vi "Periodic Tasks.vi"(8 "error in":errorcluster) -> ()   [LabVIEW 2013]
doc: "This VI runs in parallel to other tasks. It can contain as many user-defined periodic loops as you need. These can carry out PID or other sorts of timed response."
uses:
  <vilib>/Rock Robotics/SystemInterfaces/Utilities/FPGA_UtilitiesLED Source.ctl
  <vilib>/Rock Robotics/SystemInterfaces/Utilities/FPGA_UtilitiesLED State.ctl
  <vilib>/Rock Robotics/WPI/DriverStation/WPI_DriverStationRobotMode2.ctl
  <vilib>/Platform/TimedLoop/XDataNode/timing_clust.ctl
  <vilib>/Platform/TimedLoop/XDataNode/nitl_modes.ctl
  <vilib>/Platform/TimedLoop/XDataNode/wakeup.ctl
  Robot Global Data.vi
  <vilib>/Rock Robotics/WPI/Solenoid/Deprecated/WPI_SolenoidSetBool.vi
  <vilib>/addons/control/pid/pid.llb/PID (DBL).vi
  <vilib>/Rock Robotics/WPI/Compressor/WPI_CompressorGetSetRefNum.vi
  <vilib>/Platform/TimedLoop/XDataNode/XDataNode.xnode
  <vilib>/Platform/TimedLoop/XDataNode/XDNodeRunTimeDep.lvlib
  <vilib>/addons/control/pid/NI_PID_pid.lvlib
  <vilib>/addons/control/pid/pid.llb/PID Control Input Filter (DBL).vi
  Encoder Values.ctl
panel:
  in  "Neutral Angle":dbl=25.8
  in  "Feed Angle":dbl=20.0
  in  "Full Court Angle":dbl=25.8
  in  "Pyramid Angle":dbl=31.0
  in  "Vision Angle":dbl=24.5
  in  "Full Court Main RPM":dbl=4000.0
  in  "Full Court Pre RPM":dbl=3500.0
  in  "Pyramid Main RPM":dbl=4000.0
  in  "Pyramid Pre RPM":dbl=3500.0
  in  "Vision Main RPM":dbl=4000.0
  in  "Vision Pre RPM":dbl=3500.0
  in  "Elevator Enabled":bool=TRUE
  in  "Two Disc Loading":bool=TRUE
  in  "Load Reverse Enabled":bool=TRUE
  in  "Load Roller Delay (ms)":dbl=250.0
  in  "Load Exit Delay (ms)":dbl=1000.0
  in  "Shoot Exit Delay (ms)":dbl=200.0
  out "RPM Ready":bool
  out "Elevator Neutral Enabled":bool
  out "Neutral Angle Ready":bool
  out "Feed Angle Ready":bool
  out "Auto Angle Enabled":bool
  in  "Elevator Angle":dbl
  in  "Elevator Pot Voltage":dbl
  out "Shoot Angle Ready":bool
  in  "Shooter Pre RPM":dbl
  in  "Shooter Main RPM":dbl
  in  "Shooter Pre Output":dbl
  in  "Shooter Main Output":dbl
  # "don't stop wheels before disc exits shooter"
  # "don't stop rollers before disc reaches hopper"
  # "reverse rollers to push discs\n(ensures ramp can lower in time)"
  # "reverse rollers to keep discs out\n(as opposed to simply stopping)"
  # "when IRs see 2 discs, reverse right roller"
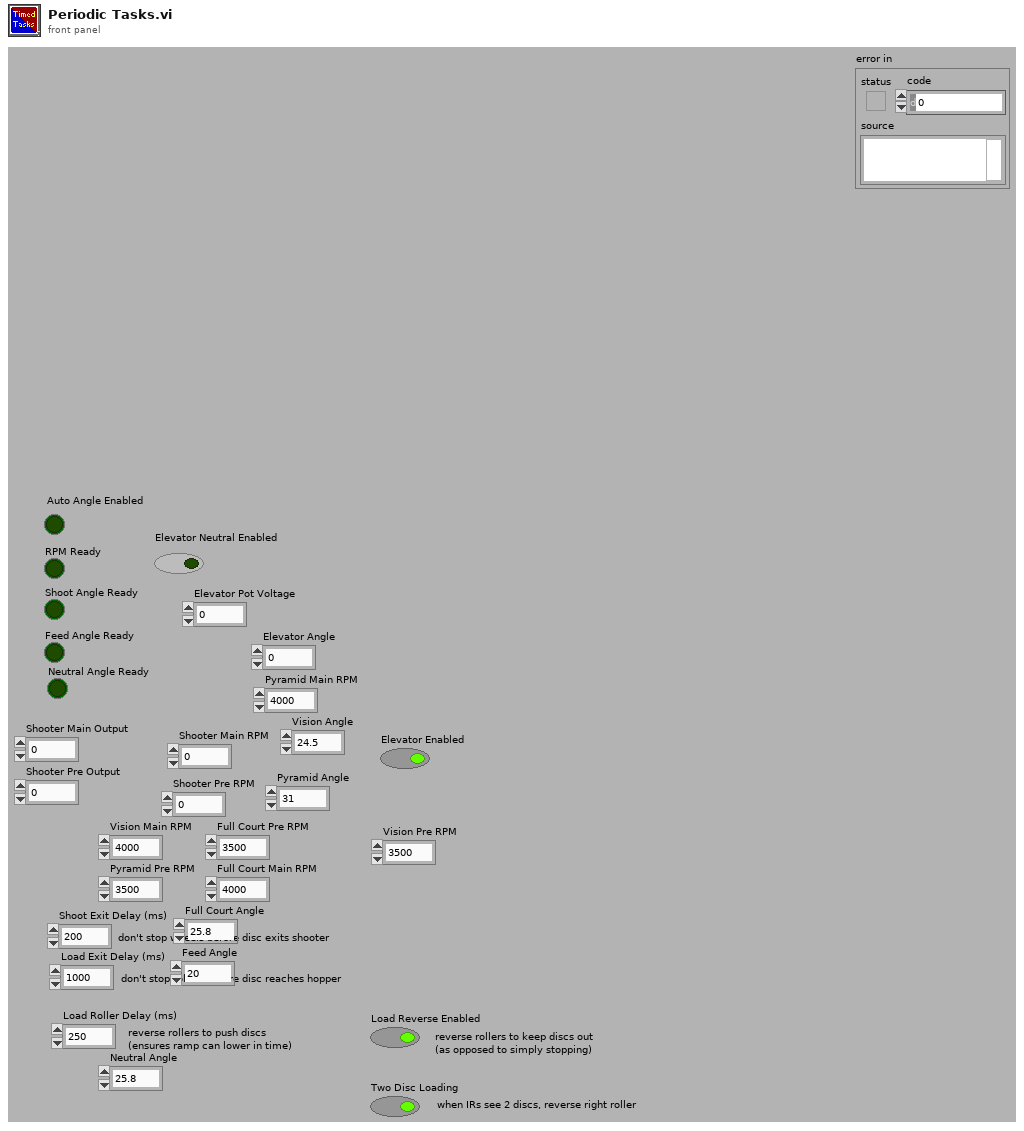
[diagram p1: front panel]
types:
  T1 = typedef "WPI_DriverStationRobotMode2.ctl" = enum16{"Autonomous Disabled", "Autonomous Enabled", "Teleop Disabled", "Teleop Enabled", "Timeout", "Finish", "Test Disabled", "Test Enabled"}
  T2 = enum16{"Vision", "Feed", "Pyramid", "Full Court"}
  T3 = cluster{"proportional gain (Kc)":dbl, "integral time (Ti, min)":dbl, "derivative time (Td, min)":dbl}
  T4 = typedef "Shoot Location.ctl" = enum16{"Vision", "Front", "Front Corner", "Back Corner", "Half Court", "Full Court", "Pyramid"}
  T5 = typedef "Autonomous Commands.ctl" = cluster{"Load":bool, "Warmup":bool, "Low Gear":bool, "Shoot Angle":dbl, "Azimuth":bool, "Elevator":bool, "Neutral Angle":dbl, "Two Discs":bool, "Shoot":bool}
  T6 = enum16{"Wait", "Adjust Angle", "Warmup Shooter", "Fire", "Feeding", "Neutral Angle"}
  T7 = typedef "XDNodeRunTimeDep.lvlib/timing_clust.ctl" = cluster{"Expected End [f-1]":u64, "Actual End [f-1]":u64, "Finished Late? [f-1]":bool, "Expected End [i-1]":u64, "Actual End [i-1]":u64, "Finished Late? [i-1]":bool, "Expected Start [i]":u64, "Actual Start [i]":u64, "Expected Start [f]":u64, "Actual Start [f]":u64, "Source Name":string, "Structure Name":string, "Period":i64, "Deadline":i64, "Offset":i64, "Start":i64, "Priority":i32, "Timeout":i32, "Mode":T8, "Wakeup Reason":T9, "Error":errorcluster, "Source Type":string, "Secondary Source Type":string, "Global End Time":u64, "Global Start Time":u64, "Frame Duration":u64, "Iteration Duration":u64, "Assigned CPU":i32, "I/O Scan Engine Mode":u32}
  T8 = typedef "XDNodeRunTimeDep.lvlib/nitl_modes.ctl" = enum32{"No Change", "Process missed periods, maintain original phase", "Discard missed periods, maintain original phase", "Process missed periods, ignore original phase", "Discard missed periods, ignore original phase"}
  T9 = typedef "XDNodeRunTimeDep.lvlib/wakeup.ctl" = enum32{"Normal", "Aborted", "Asynchronous wakeup", "Timing source error", "Timed loop error", "Timeout"}
  T10 = typedef "WPI_JoystickButtonState.ctl" = cluster{"Button 1":bool, "Button 2":bool, "Button 3":bool, "Button 4":bool, "Button 5":bool, "Button 6":bool, "Button 7":bool, "Button 8":bool, "Button 9":bool, "Button 10":bool, "Button 11":bool, "Button 12":bool}
  T11 = cluster{"Driver Axes":cluster{"axis 1 (x)":dbl, "axis 2 (y)":dbl, "axis 3 (throttle)":dbl, "axis 4":dbl, "axis 5":dbl, "axis 6":dbl}, "Driver Buttons":T10, "Manipulator Axes":cluster{"axis 1 (x)":dbl, "axis 2 (y)":dbl, "axis 3 (throttle)":dbl, "axis 4":dbl, "axis 5":dbl, "axis 6":dbl}, "Manipulator Buttons":T10}
  T12 = typedef "UDP Dashboard Packet.ctl" = cluster{"Feed Angle":dbl, "Neutral Angle":dbl, "Autonomous Setpoints":T13, "Auto Shift":T14, "Elevator Angle Offset":dbl, "Potentiometer Angle":cluster{"Pot M":dbl, "Pot B":dbl}, "Shoot Setpoints":cluster{"Vision":T15, "Back Corner":T15, "Front":T15, "Front Corner":T15, "Half Court":T15, "Full Court":T15, "Pyramid":T15}, "Halo Drive":T16, "Auto Speed Constants":T17, "Shooting Delays":cluster{"Unjam On":dbl, "Unjam Off":dbl, "Flipper On":dbl, "Flipper Off":dbl, "Hopper Up":dbl}, "Left Roller Pwr":dbl, "Right Roller Pwr":dbl, "Elevator PID Gains":cluster{"proportional gain (Kc)":dbl, "integral time (Ti, min)":dbl, "derivative time (Td, min)":dbl}, "Elevator PID Output Range":cluster{"output high":dbl, "output low":dbl}, "Elevator Angle Tolerance":dbl, "Toggle Ears Delay":dbl, "Toggle Ears Distance":dbl, "Unjam Servo Angle":dbl, "Auton Steer PID gains":cluster{"proportional gain (Kc)":dbl, "integral time (Ti, min)":dbl, "derivative time (Td, min)":dbl}, "Auton Steer output range":cluster{"output high":dbl, "output low":dbl}, "Auto Reverse Speed":dbl, "Auto Stop Throttle":dbl, "Auto Stop Duration":dbl, "Spin output range":cluster{"output high":dbl, "output low":dbl}, "Spin PID gains":cluster{"proportional gain (Kc)":dbl, "integral time (Ti, min)":dbl, "derivative time (Td, min)":dbl}, "Auto-Center Line":T18, "Auton Distance PID gains Low Gear":cluster{"proportional gain (Kc)":dbl, "integral time (Ti, min)":dbl, "derivative time (Td, min)":dbl}, "Auton Distance output range":cluster{"output high":dbl, "output low":dbl}, "Auton Distance Threshold":dbl, "Auton Velocity Cutoff":dbl, "Auton Distance output range Center Line":cluster{"output high":dbl, "output low":dbl}, "Auton Distance PID gains High Gear":cluster{"proportional gain (Kc)":dbl, "integral time (Ti, min)":dbl, "derivative time (Td, min)":dbl}}
  T13 = typedef "Autonomous Setpoints.ctl" = cluster{"Shoot Angle 1":dbl, "Initial Delay":dbl, "Disc Count 1":dbl, "Shoot Time 1":dbl, "Distance 1":dbl, "Two Disc Distance 1":dbl, "Distance 2":dbl, "Two Disc Distance 2":dbl, "Distance 3":dbl, "Two Disc Distance 3":dbl, "Shoot Angle 3":dbl, "Disc Count 3":dbl, "Shoot Time 3":dbl, "Distance 4":dbl, "Two Disc Distance 4":dbl, "Low Gear":bool, "Shoot 1 Post Delay":dbl}
  T14 = typedef "Auto Shift Settings.ctl" = cluster{"Enabled":bool, "Upshift Speed":dbl, "Downshift Speed":dbl, "Upshift Throttle":dbl, "Turn Power Diff":dbl, "Motor Limit":dbl, "Encoder Limit":dbl}
  T15 = typedef "Shoot Profile.ctl" = cluster{"Pre RPM":dbl, "Main RPM":dbl, "Angle":dbl}
  T16 = typedef "Halo Drive.ctl" = cluster{"Gains":cluster{"Quickturn_Sens_Low":dbl, "Quickturn_Sens_High":dbl, "Speedturn_Sens_Low":dbl, "Speedturn_Sens_High":dbl}, "QuickTurn Const":dbl, "Loading Throttle Limit":dbl}
  T17 = typedef "Auto Speed Constants.ctl" = cluster{"Slowing Distance":dbl, "High Speed":dbl, "Rampup Time":dbl, "Low Speed":dbl, "High Speed (Reverse)":dbl}
  T18 = typedef "Autonomous Center Line Setpoints.ctl" = cluster{"Arc Turn x-axis":dbl, "Arc Turn y-axis":dbl, "Arc Turn Distance":dbl, "Distance 1":dbl, "Two Disc Distance 1":dbl, "Distance 2":dbl, "Two Disc Distance 2":dbl, "Spin Angle":dbl, "Spin Angle tolerance":dbl, "Spin y-axis":dbl, "Spin Distance":dbl, "Center Line Enabled":bool, "Distance 3":dbl, "Two Disc Distance 3":dbl, "Spin Angle 2":dbl, "Spin Angle tolerance 2":dbl, "Spin y-axis 2":dbl, "Spin Distance 2":dbl, "Shoot Angle 1":dbl, "Disc Count 1":dbl, "Shoot Time 1":dbl, "Shoot Angle 3":dbl, "Disc Count 3":dbl, "Shoot Time 3":dbl, "Low Gear":bool}
  T19 = typedef "FPGA_UtilitiesLED State.ctl" = enum16{"Off", "On", "Toggle"}
  T20 = typedef "FPGA_UtilitiesLED Source.ctl" = enum16{"User LED", "FPGA LED"}
  T21 = typedef "WPI_CompressorDevRef.ctl" = cluster{"DevStatus":errorcluster, "DigitalInputDevRef":T22, "RelayDevRef":T25}
  T22 = typedef "WPI_DigitalInputDevRef.ctl" = cluster{"DevStatus":errorcluster, "DIO Channel":T23, "Digital Module":T24}
  T23 = typedef "FPGA_DIOChannel.ctl" = enum8{"DIO 1", "DIO 2", "DIO 3", "DIO 4", "DIO 5", "DIO 6", "DIO 7", "DIO 8", "DIO 9", "DIO 10", "DIO 11", "DIO 12", "DIO 13", "DIO 14", "Invalid"}
  T24 = typedef "FPGA_TypedefDigitalModule.ctl" = enum16{"Digital Module 1", "Digital Module 2"}
  T25 = typedef "WPI_RelayDevRef.ctl" = cluster{"DevStatus":errorcluster, "Relay Channel":T26, "Digital Module":T24, "Relay Direction":T27}
  T26 = typedef "FPGA_DIORelayChannel.ctl" = enum8{"Relay 1", "Relay 2", "Relay 3", "Relay 4", "Relay 5", "Relay 6", "Relay 7", "Relay 8", "Invalid"}
  T27 = typedef "WPI_RelayDirection.ctl" = enum16{"Both directions", "Forward only", "Reverse only"}
  T28 = typedef "WPI_GyroDevRef.ctl" = cluster{"DevStatus":errorcluster, "Analog Module":T29, "Analog Channel":T30, "Offset":dbl, "Gain (VoltsPerDegree/Second)":dbl}
  T29 = typedef "FPGA_TypedefAnalogModule.ctl" = enum16{"Analog Module 1", "Analog Module 2"}
  T30 = typedef "FPGA_AIChannel.ctl" = enum8{"AI 1", "AI 2", "AI 3", "AI 4", "AI 5", "AI 6", "AI 7", "AI 8", "Invalid"}
  T31 = typedef "WPI_EncoderDevRef.ctl" = cluster{"DevStatus":errorcluster, "EncoderIndex":T32, "CounterIndex":T33, "DistancePerCount":dbl, "Decoding Type":T34}
  T32 = typedef "FPGA_EncoderIdx.ctl" = enum8{"Enc 0", "Enc 1", "Enc 2", "Enc 3", "Invalid"}
  T33 = typedef "FPGA_CounterCtrSystemIndex.ctl" = enum8{"Ctr 0", "Ctr 1", "Ctr 2", "Ctr 3", "Ctr 4", "Ctr 5", "Ctr 6", "Ctr 7", "Invalid"}
  T34 = typedef "WPI_EncoderType.ctl" = enum16{"1x", "2x", "4x"}
  T35 = typedef "WPI_MotorControlDeviceRef.ctl" = cluster{"DeviceStatus":errorcluster, "Type":enum16{"PWM", "CAN"}, "PWM":cluster{"Digital Module":T24, "PWM Channel":T36, "DeadBand":T37}, "CAN":cluster{"Device Number":u8, "Control Mode":T38, "Semaphore":T39, "Max Vout":dbl}, "Invert":bool, "TransformRef":T40, "InvTransformRef":T40}
  T36 = typedef "FPGA_DIOPWMChannel.ctl" = enum8{"PWM 1", "PWM 2", "PWM 3", "PWM 4", "PWM 5", "PWM 6", "PWM 7", "PWM 8", "PWM 9", "PWM 10", "Invalid"}
  T37 = typedef "WPI_PWMDeadband.ctl" = cluster{"Name":string, "maxPositivePwm":i32, "minPositivePwm":i32, "centerPwm":i32, "maxNegativePwm":i32, "minNegativePwm":i32, "angularRange":u16}
  T38 = typedef "WPI_CANJaguar_ControlMode.ctl" = enum8{"Percent VBus", "Current", "Speed", "Position", "Voltage"}
  T39 = typedef "Semaphore RefNum" = refnum<k1>
  T40 = typedef "WPI_PWMTransform_ConPane.ctl" = refnum<vi>
  T41 = typedef "Encoder Values.ctl" = cluster{"Left Dist":dbl, "Left Speed":dbl, "Right Dist":dbl, "Right Speed":dbl, "Left Ticks":dbl, "Right Ticks":dbl, "Avg Distance":dbl, "Avg Speed":dbl}
  T42 = cluster{"Wheel IR 1":bool, "Wheel IR 2":bool, "Disc IR Front":bool, "Disc IR Front 2":bool, "Disc IR Hopper":bool, "Disc IR Shooter":bool}
  T43 = cluster{"axis 1 (x)":dbl, "axis 2 (y)":dbl, "axis 3 (throttle)":dbl, "axis 4":dbl, "axis 5":dbl, "axis 6":dbl}
  T44 = cluster{"Manual Unjam":bool, "Manual Flipper":bool}
  T45 = cluster{"Unjam On":dbl, "Unjam Off":dbl, "Flipper On":dbl, "Flipper Off":dbl, "Hopper Up":dbl}
  T46 = typedef "WPI_ServoDeviceRef.ctl" = cluster{"DeviceStatus":errorcluster, "Digital Module":T24, "PWM Channel":T36, "DeadBand":T37}
  T47 = cluster{"Throttle":dbl, "Wheel":dbl, "Right Motor":dbl, "Left Motor":dbl}
  T48 = typedef "WPI_SolenoidDevRef.ctl" = cluster{"DevStatus":errorcluster, "Solenoid Module":T49, "Forward Solenoid Channel":T50, "Reverse Solenoid Channel":T50}
  T49 = typedef "FPGA_TypedefSolenoidModule.ctl" = enum16{"Solenoid Module 1", "Solenoid Module 2"}
  T50 = typedef "WPI_SolenoidChannel.ctl" = enum8{"Solenoid 1", "Solenoid 2", "Solenoid 3", "Solenoid 4", "Solenoid 5", "Solenoid 6", "Solenoid 7", "Solenoid 8", "Invalid"}
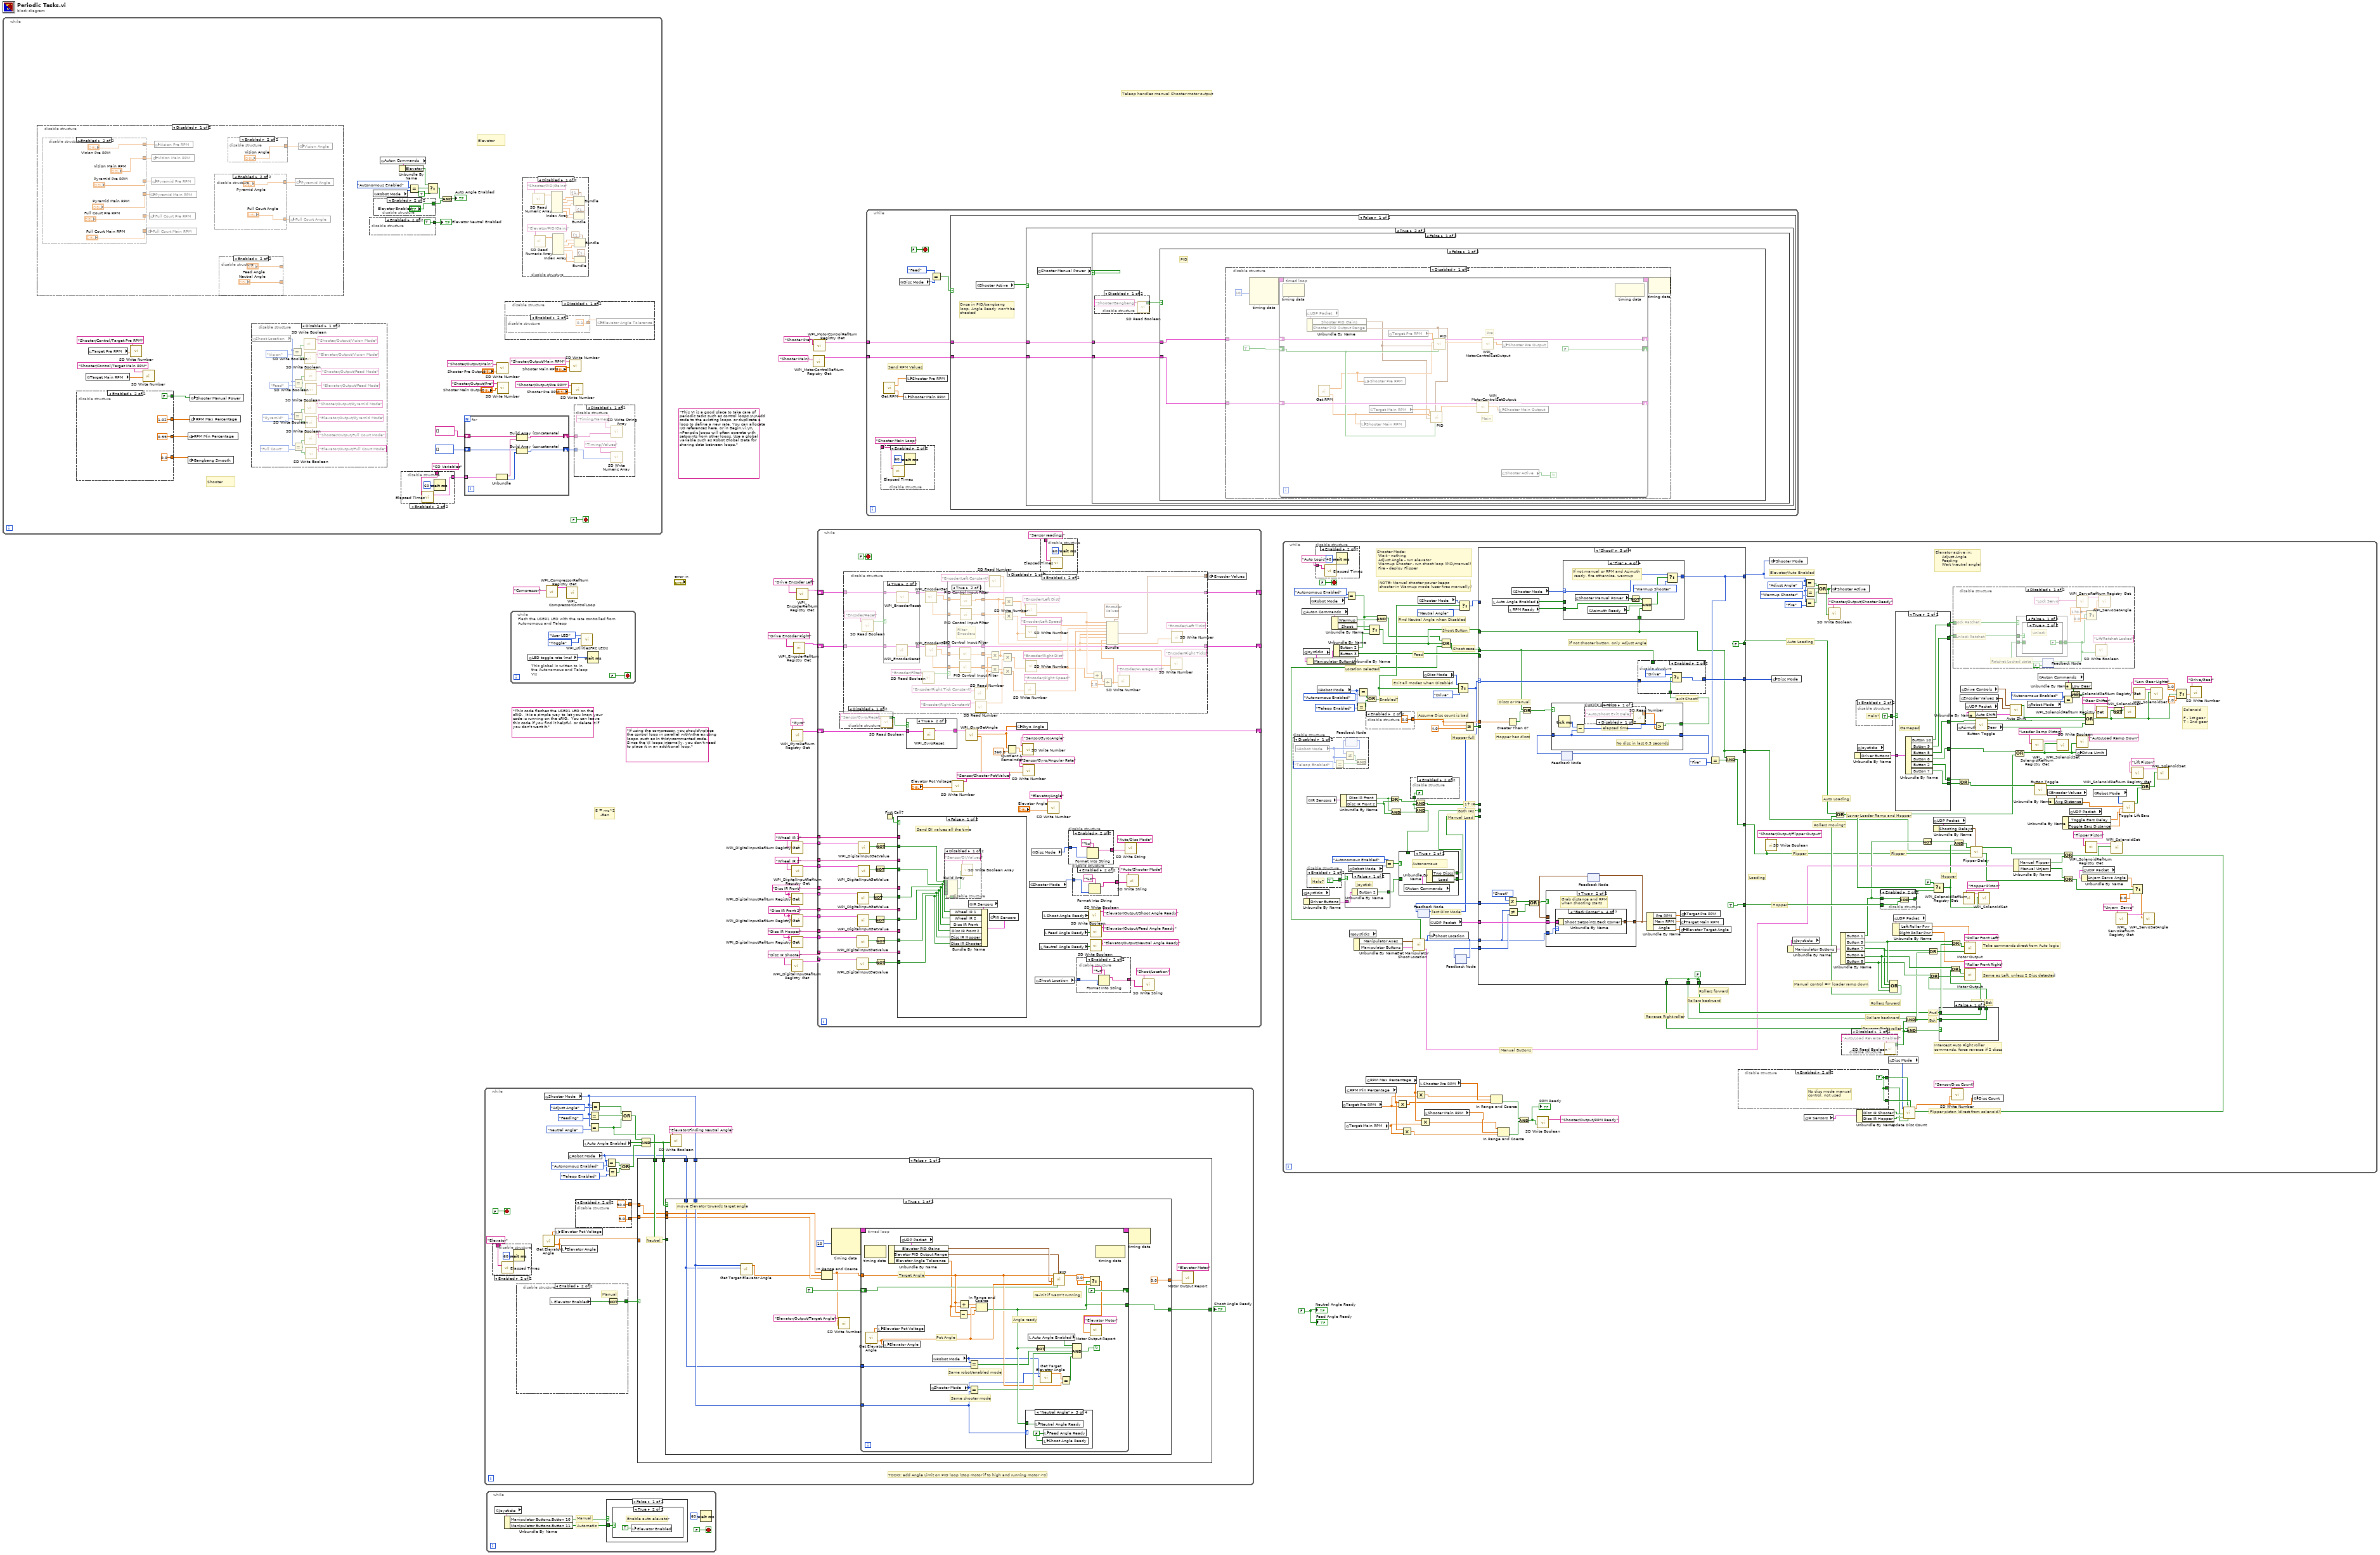
[diagram p0: block diagram]
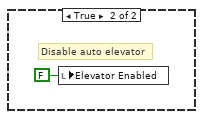
[diagram p3: hidden frame]
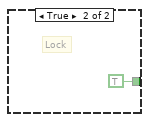
[diagram p5: hidden frame]
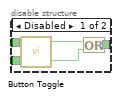
[diagram p7: hidden frame]
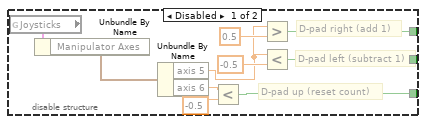
[diagram p9: hidden frame]
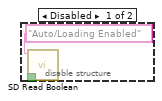
[diagram p10: hidden frame]
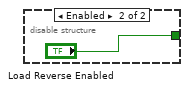
[diagram p11: hidden frame]
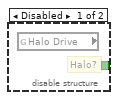
[diagram p12: hidden frame]
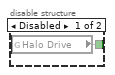
[diagram p13: hidden frame]
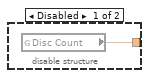
[diagram p15: hidden frame]
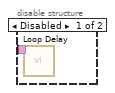
[diagram p16: hidden frame]
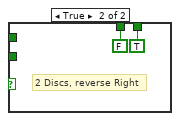
[diagram p17: hidden frame]
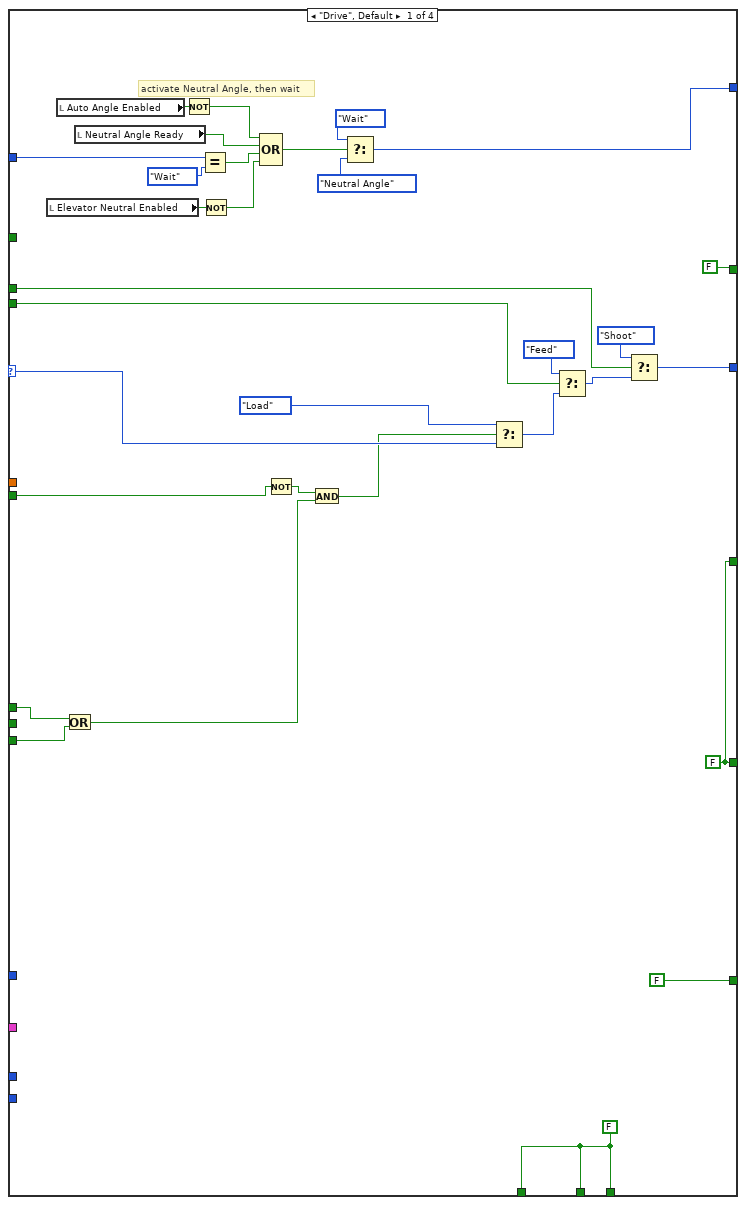
[diagram p18: hidden frame]
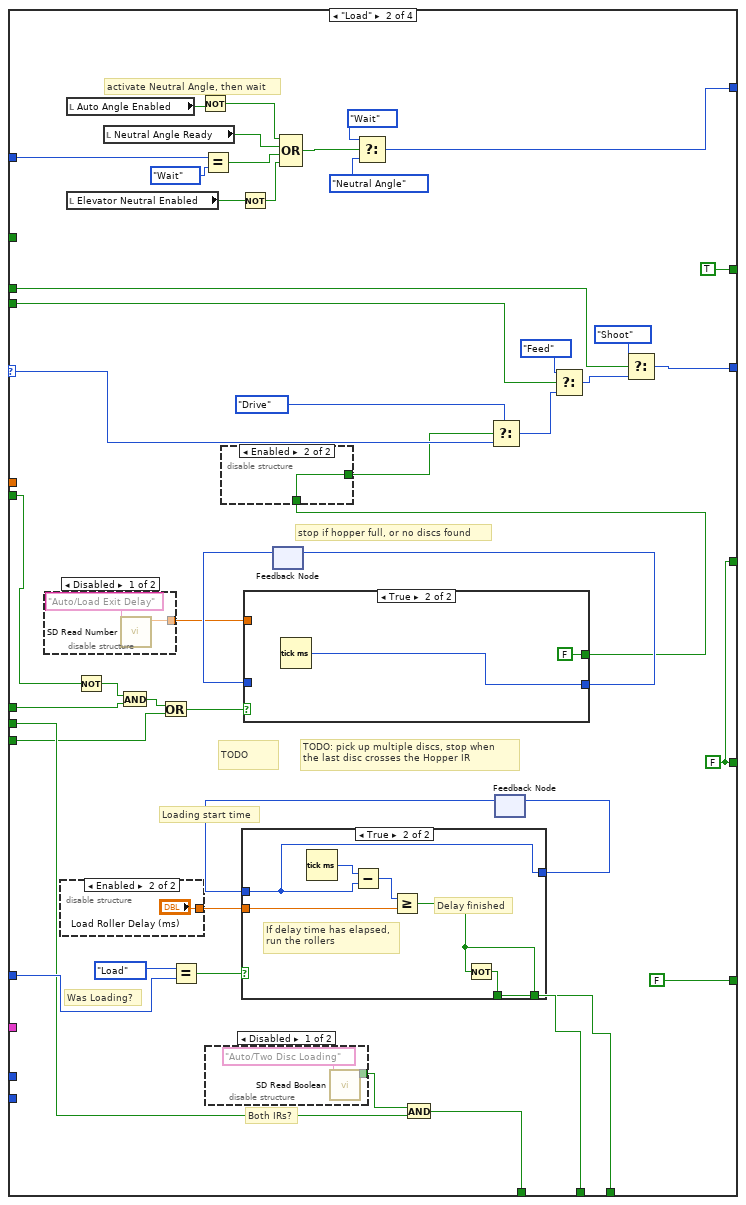
[diagram p19: hidden frame]
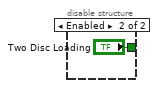
[diagram p20: hidden frame]
diagram:
  w1 = FALSE
  w2 = "Disc IR Shooter" ("refnum name")
  w6 = "Disc IR Hopper" ("refnum name")
  w5 = "Disc IR Front 2" ("refnum name")
  w4 = "Disc IR Front" ("refnum name")
  w11 = "Wheel IR 2" ("refnum name")
  w12 = "Wheel IR 1" ("refnum name")
  (unwired) "If using the compressor, you should\nplace the control loop in parallel with\nthe existing loops, such as in this\ncommented code. Since the VI loops internally, you don't need to place it in an additional loop."
  (unwired) "This code flashes the USER1 LED on the cRIO.  It is a simple way to let you know your code is running on the cRIO.  You can leave this code if you find it helpful, or delete it if you don't want it."
  (unwired) "This VI is a good place to take care of periodic tasks such as control loops.\n\nAdd code to the existing loops, or duplicate a loop to define a new rate. You can allocate I/O references here, or in Begin.vi.\n\nPeriodic loops will often operate with setpoints from other loops. Use a global variable such as Robot Global Data for sharing data between loops."
  # "Teleop handles manual Shooter motor output"
  # "E = mc^2\n    -Ben"
  n1 = while {
    stop <- FALSE stop-if-true
    # "Elevator"
    # "Shooter"
    n2 = disable-structure shown="Disabled" {
      frame Disabled {
        n3 = disable-structure shown="Enabled" {
          disable-tunnel: [w111 "Vision Pre RPM"] -> w88
          disable-tunnel: [w108 "Vision Main RPM"] -> w87
          disable-tunnel: [w107 "Pyramid Pre RPM"] -> w86
          disable-tunnel: [w104 "Pyramid Main RPM"] -> w85
          disable-tunnel: [w103 "Full Court Pre RPM"] -> w84
          disable-tunnel: [w100 "Full Court Main RPM"] -> w83
          frame Disabled {
            n4 = call <vilib>:"SD Read Number.vi"("Name"="Shooter/Control/Full Court Main RPM") -> ("Numeric"=w100:dbl)  [unwired: 8 in, 2 out]
            n5 = call <vilib>:"SD Read Number.vi"("Name"="Shooter/Control/Full Court Pre RPM") -> ("Numeric"=w103:dbl)  [unwired: 8 in, 2 out]
            n6 = call <vilib>:"SD Read Number.vi"("Name"="Shooter/Control/Vision Main RPM") -> ("Numeric"=w108:dbl)  [unwired: 8 in, 2 out]
            n7 = call <vilib>:"SD Read Number.vi"("Name"="Shooter/Control/Pyramid Pre RPM") -> ("Numeric"=w107:dbl)  [unwired: 8 in, 2 out]
            n8 = call <vilib>:"SD Read Number.vi"("Name"="Shooter/Control/Pyramid Main RPM") -> ("Numeric"=w104:dbl)  [unwired: 8 in, 2 out]
            n9 = call <vilib>:"SD Read Number.vi"("Name"="Shooter/Control/Vision Pre RPM") -> ("Numeric"=w111:dbl)  [unwired: 8 in, 2 out]
          }
          frame Enabled {
          }
        }
        n10 = global write "Robot Global Data.vi" "Full Court Main RPM"(w83) -> ()
        n11 = global write "Robot Global Data.vi" "Full Court Pre RPM"(w84) -> ()
        n12 = global write "Robot Global Data.vi" "Pyramid Main RPM"(w85) -> ()
        n13 = global write "Robot Global Data.vi" "Pyramid Pre RPM"(w86) -> ()
        n14 = global write "Robot Global Data.vi" "Vision Main RPM"(w87) -> ()
        n15 = global write "Robot Global Data.vi" "Vision Pre RPM"(w88) -> ()
        n16 = disable-structure shown="Enabled" {
          disable-tunnel: [w96 "Pyramid Angle"] -> w81
          disable-tunnel: [w95 "Full Court Angle"] -> w80
          frame Disabled {
            n17 = call <vilib>:"SD Read Number.vi"("Name"="Elevator/Full Court Angle") -> ("Numeric"=w95:dbl)  [unwired: 8 in, 2 out]
            n18 = call <vilib>:"SD Read Number.vi"("Name"="Elevator/Pyramid Angle") -> ("Numeric"=w96:dbl)  [unwired: 8 in, 2 out]
          }
          frame Enabled {
          }
        }
        n19 = disable-structure shown="Enabled" {
          disable-tunnel: [w121 "Feed Angle"] -> w90
          disable-tunnel: [w118 "Neutral Angle"] -> w89
          frame Disabled {
            n20 = call <vilib>:"SD Read Number.vi"("Name"="Elevator/Feed Angle") -> ("Numeric"=w121:dbl)  [unwired: 8 in, 2 out]
            n21 = call <vilib>:"SD Read Number.vi"("Name"="Elevator/Neutral Angle") -> ("Numeric"=w118:dbl)  [unwired: 8 in, 2 out]
          }
          frame Enabled {
          }
        }
        n22 = disable-structure shown="Enabled" {
          disable-tunnel: [w92 "Vision Angle"] -> w82
          frame Disabled {
            n23 = call <vilib>:"SD Read Number.vi"("Name"="Elevator/Vision Angle") -> ("Numeric"=w92:dbl)  [unwired: 8 in, 2 out]
          }
          frame Enabled {
          }
        }
        n24 = global write "Robot Global Data.vi" "Full Court Angle"(w80) -> ()
        n25 = global write "Robot Global Data.vi" "Pyramid Angle"(w81) -> ()
        n26 = global write "Robot Global Data.vi" "Vision Angle"(w82) -> ()
      }
      frame Enabled {
      }
    }
    n27 = disable-structure shown="Enabled" {
      disable-tunnel: [w136 0.0 ("Bangbang Smooth")] -> w52
      disable-tunnel: [w134 1.02 ("RPM Max Percentage")] -> w50
      disable-tunnel: [w133 0.99 ("RPM Min Percentage")] -> w49
      disable-tunnel: [w130 FALSE ("Shooter Manual Power")] -> w48
      frame Disabled {
        n28 = call <vilib>:"SD Read Number.vi"("Name"="Shooter/Control/RPM Min Percentage") -> ("Numeric"=w133:dbl)  [unwired: 8 in, 2 out]
        n29 = call <vilib>:"SD Read Number.vi"("Name"="Shooter/Bangbang Smooth") -> ("Numeric"=w136:dbl)  [unwired: 8 in, 2 out]
        n30 = call <vilib>:"SD Read Number.vi"("Name"="Shooter/Control/RPM Max Percentage") -> ("Numeric"=w134:dbl)  [unwired: 8 in, 2 out]
        n31 = call <vilib>:"SD Read Boolean.vi"("Name"="Shooter/Manual Power") -> ("Boolean"=w130:bool)  [unwired: 8 in, 2 out]
      }
      frame Enabled {
      }
    }
    n32 = global read "Robot Global Data.vi" "Target Main RPM"() -> (w27:dbl)
    n33 = global read "Robot Global Data.vi" "Target Pre RPM"() -> (w26:dbl)
    n34 = call <vilib>:"SD Write Number.vi"("Numeric"=w26, "Name"="Shooter/Control/Target Pre RPM") -> ()  [unwired: 8 in, 2 out]
    n35 = call <vilib>:"SD Write Number.vi"("Numeric"=w27, "Name"="Shooter/Control/Target Main RPM") -> ()  [unwired: 8 in, 2 out]
    n36 = global write "Robot Global Data.vi" "RPM Min Percentage"(w49) -> ()
    n37 = global write "Robot Global Data.vi" "Bangbang Smooth"(w52) -> ()
    n38 = global write "Robot Global Data.vi" "RPM Max Percentage"(w50) -> ()
    n39 = global write "Robot Global Data.vi" "Shooter Manual Power"(w48) -> ()
    n40 = disable-structure shown="Disabled" {
      frame Disabled {
        n41 = global read "Robot Global Data.vi" "Shoot Location"() -> (w67:T4)
        n42 = Equal?(x=w67, y=T2."Vision") -> (x = y?=w77:bool)
        n43 = Equal?(x=w67, y=T2."Pyramid") -> (x = y?=w71:bool)
        n44 = Equal?(x=w67, y=T2."Feed") -> (x = y?=w76:bool)
        n45 = Equal?(x=w67, y=T2."Full Court") -> (x = y?=w70:bool)
        n46 = call <vilib>:"SD Write Boolean.vi"("Boolean"=w77, "Name"="Shooter/Output/Vision Mode") -> ()  [unwired: 8 in, 2 out]
        n47 = call <vilib>:"SD Write Boolean.vi"("Boolean"=w77, "Name"="Elevator/Output/Vision Mode") -> ()  [unwired: 8 in, 2 out]
        n48 = call <vilib>:"SD Write Boolean.vi"("Boolean"=w71, "Name"="Shooter/Output/Pyramid Mode") -> ()  [unwired: 8 in, 2 out]
        n49 = call <vilib>:"SD Write Boolean.vi"("Boolean"=w76, "Name"="Shooter/Output/Feed Mode") -> ()  [unwired: 8 in, 2 out]
        n50 = call <vilib>:"SD Write Boolean.vi"("Boolean"=w70, "Name"="Shooter/Output/Full Court Mode") -> ()  [unwired: 8 in, 2 out]
        n51 = call <vilib>:"SD Write Boolean.vi"("Boolean"=w71, "Name"="Elevator/Output/Pyramid Mode") -> ()  [unwired: 8 in, 2 out]
        n52 = call <vilib>:"SD Write Boolean.vi"("Boolean"=w76, "Name"="Elevator/Output/Feed Mode") -> ()  [unwired: 8 in, 2 out]
        n53 = call <vilib>:"SD Write Boolean.vi"("Boolean"=w70, "Name"="Elevator/Output/Full Court Mode") -> ()  [unwired: 8 in, 2 out]
      }
      frame Enabled {
      }
    }
    n54 = disable-structure shown="Enabled" {
      disable-tunnel: [w127 TRUE ("Elevator Neutral Enabled")] -> w37
      frame Disabled {
        n55 = call <vilib>:"SD Read Boolean.vi"("Name"="Elevator/Neutral Enabled") -> ("Boolean"=w127:bool)  [unwired: 8 in, 2 out]
      }
      frame Enabled {
      }
    }
    "Elevator Neutral Enabled" <- w37
    n56 = global read "Robot Global Data.vi" "Robot Mode"() -> (w33:T1)
    n57 = disable-structure shown="Enabled" {
      disable-tunnel: [w124 "Elevator Enabled"] -> w35
      frame Disabled {
        n58 = call <vilib>:"SD Read Boolean.vi"("Name"="Elevator/Auto Enabled") -> ("Boolean"=w124:bool)  [unwired: 8 in, 2 out]
      }
      frame Enabled {
      }
    }
    n59 = global read "Robot Global Data.vi" "Auton Commands"() -> (w36:T5)
    n60 = Unbundle By Name(w36) -> ("Elevator"=w30:bool)
    n61 = disable-structure shown="Enabled" {
      disable-tunnel: "SD Variables" ("Call Name") -> [w165 w167]
      disable-tunnel: [w164 w166] -> w38
      frame Disabled {
        n62 = call "Loop Delay.vi"("Loop Name"=w165) -> ("Timings"=w164:cluster{"Call Name":string, "Delta (ms)":u32}[])  [unwired: 10 in]
      }
      frame Enabled {
        n63 = call "Elapsed Times.vi"("Call Name"=w167) -> ("Timings"=w166:cluster{"Call Name":string, "Delta (ms)":u32}[])  [unwired: 2 in]
        n64 = Wait (ms)(milliseconds to wait=u32 60 ("t")) -> ()  [unwired: 1 out]
      }
    }
    n65 = Equal?(x=WPI_DriverStationRobotMode2."Autonomous Enabled", y=w33) -> (x = y?=w31:bool)
    n66 = Select(t=w30, s=w31, f=TRUE) -> (s? t:f=w29:bool)
    n67 = And(x=w29, y=w35) -> (x .and. y?=→"Auto Angle Enabled":bool)
    n68 = for {
      tunnel: w38 -> [w175] mode=indexing
      shift-right: [w170] -> w55
      shift-left: string[] [] ("appended array") -> [w171]
      shift-right: [w169] -> w54
      shift-left: u32[] [] ("appended array") -> [w172]
      n69 = Unbundle(w175) -> ("Call Name"=w174:string, "Delta (ms)"=w173:u32)
      n70 = Build Array (concatenate)(w171, w174) -> (w170:string[])
      n71 = Build Array (concatenate)(w172, w173) -> (w169:u32[])
    }
    n72 = call <vilib>:"SD Write Number.vi"("Numeric"="Shooter Pre Output", "Name"="Shooter/Output/Main") -> ()  [unwired: 8 in, 2 out]
    n73 = call <vilib>:"SD Write Number.vi"("Numeric"="Shooter Main Output", "Name"="Shooter/Output/Pre") -> ()  [unwired: 8 in, 2 out]
    n74 = disable-structure shown="Disabled" {
      frame Disabled {
        n75 = disable-structure shown="Enabled" {
          disable-tunnel: [w60 0.1 ("Elevator Angle Tolerance")] -> w59
          frame Disabled {
            n76 = call <vilib>:"SD Read Number.vi"("Name"="Elevator/Control/Angle Tolerance") -> ("Numeric"=w60:dbl)  [unwired: 8 in, 2 out]
          }
          frame Enabled {
          }
        }
        n77 = global write "Robot Global Data.vi" "Elevator Angle Tolerance"(w59) -> ()
      }
      frame Enabled {
      }
    }
    n78 = disable-structure shown="Disabled" {
      frame Disabled {
        n79 = call <vilib>:"SD Read Numeric Array.vi"("Name"="Shooter/PID/Gains") -> ("Numeric Array"=w157:dbl[])  [unwired: 8 in, 2 out]
        n80 = call <vilib>:"SD Read Numeric Array.vi"("Name"="Elevator/PID/Gains") -> ("Numeric Array"=w148:dbl[])  [unwired: 8 in, 2 out]
        n81 = Index Array(array=w157) -> (element #1=w156:dbl, element #2=w155:dbl, element #3=w154:dbl, element #4=w143:dbl, element #5=w142:dbl)  [unwired: 5 in]
        n82 = Index Array(array=w148) -> (element #1=w149:dbl, element #2=w150:dbl, element #3=w151:dbl, element #4=w145:dbl, element #5=w144:dbl)  [unwired: 5 in]
        n83 = Bundle(cluster=cluster{"output high":dbl, "output low":dbl} {"output high"=100.0, "output low"=-100.0} ("output range"), "output high"=w143, "output low"=w142) -> ()  [unwired: 1 out]
        n84 = Bundle(cluster=T3 {"proportional gain (Kc)"=1.0, "integral time (Ti, min)"=0.01, "derivative time (Td, min)"=0.0} ("PID gains"), "proportional gain (Kc)"=w156, "integral time (Ti, min)"=w155, "derivative time (Td, min)"=w154) -> ()  [unwired: 1 out]
        n85 = Bundle(cluster=cluster{"output high":dbl, "output low":dbl} {"output high"=100.0, "output low"=-100.0} ("output range"), "output high"=w145, "output low"=w144) -> ()  [unwired: 1 out]
        n86 = Bundle(cluster=T3 {"proportional gain (Kc)"=1.0, "integral time (Ti, min)"=0.01, "derivative time (Td, min)"=0.0} ("PID gains"), "proportional gain (Kc)"=w149, "integral time (Ti, min)"=w150, "derivative time (Td, min)"=w151) -> ()  [unwired: 1 out]
      }
      frame Enabled {
      }
    }
    n87 = call <vilib>:"SD Write Number.vi"("Numeric"="Shooter Main RPM", "Name"="Shooter/Output/Main RPM") -> ()  [unwired: 8 in, 2 out]
    n88 = call <vilib>:"SD Write Number.vi"("Numeric"="Shooter Pre RPM", "Name"="Shooter/Output/Pre RPM") -> ()  [unwired: 8 in, 2 out]
    n89 = disable-structure shown="Disabled" {
      disable-tunnel: w55 -> [w163 _]
      disable-tunnel: w54 -> [w161 _]
      frame Disabled {
        n90 = call <vilib>:"SD Write String Array.vi"("String Array"=w163, "Name"="Timing/Names") -> ()  [unwired: 8 in, 2 out]
        n91 = call <vilib>:"SD Write Numeric Array.vi"("Numeric Array"=w161, "Name"="Timing/Values") -> ()  [unwired: 8 in, 2 out]
      }
      frame Enabled {
      }
    }
  }
  n92 = while {
    stop <- FALSE stop-if-true
    # "TODO: add Angle Limit on PID loop (stop motor if to high and running motor >0)"
    n93 = disable-structure shown="Enabled" {
      disable-tunnel: "Elevator" ("Call Name") -> [w215 w216]
      frame Disabled {
        n94 = call "Loop Delay.vi"("Loop Name"=w215) -> ()  [unwired: 10 in, 1 out]
      }
      frame Enabled {
        n95 = call "Elapsed Times.vi"("Call Name"=w216) -> ()  [unwired: 2 in, 1 out]
        n96 = Wait (ms)(milliseconds to wait=u32 60 ("t")) -> ()  [unwired: 1 out]
      }
    }
    n97 = disable-structure shown="Enabled" {
      disable-tunnel: [w202 w208] -> w198
      frame Disabled {
        # "Manual control button"
        n98 = global read "Robot Global Data.vi" "Joysticks"() -> (w200:T11)
        n99 = Unbundle By Name(w200) -> ("Manipulator Buttons.Button 10"=w202:bool, "Manipulator Buttons.Button 11"=w201:bool)
        n100 = case shown="True" w201 {
          frame False {
          }
          frame True {
            # "Enable auto elevator"
            n101 = disable-structure shown="Disabled" {
              disable-tunnel: TRUE ("Boolean") -> [w205 w206]
              frame Disabled {
                n102 = call <vilib>:"SD Write Boolean.vi"("Boolean"=w205, "Name"="Elevator/Auto Enabled") -> ()  [unwired: 8 in, 2 out]
              }
              frame Enabled {
                n103 = local write "Elevator Enabled"(w206) -> ()
              }
            }
          }
        }
      }
      frame Enabled {
        # "Manual"
        n104 = local read "Elevator Enabled"() -> (w207:bool)
        n105 = Not(x=w207) -> (.not. x?=w208:bool)
      }
    }
    n106 = call "Get Elevator Angle.vi"() -> ("Elevator Angle"=w196:dbl, "Pot Voltage"=w197:dbl)  [unwired: 2 in]
    n107 = global read "Robot Global Data.vi" "Shooter Mode"() -> (w191:T6)
    n108 = local write "Elevator Pot Voltage"(w197) -> ()
    n109 = local write "Elevator Angle"(w196) -> ()
    n110 = global read "Robot Global Data.vi" "Robot Mode"() -> (w176:T1)
    n111 = disable-structure shown="Enabled" {
      disable-tunnel: [w210 50.0 ("Numeric")] -> w195
      disable-tunnel: [w209 5.0 ("Numeric")] -> w194
      frame Disabled {
        n112 = call <vilib>:"SD Read Number.vi"("Name"="Elevator/Min Angle") -> ("Numeric"=w209:dbl)  [unwired: 8 in, 2 out]
        n113 = call <vilib>:"SD Read Number.vi"("Name"="Elevator/Max Angle") -> ("Numeric"=w210:dbl)  [unwired: 8 in, 2 out]
      }
      frame Enabled {
      }
    }
    n114 = local read "Auto Angle Enabled"() -> (w187:bool)
    n115 = Equal?(x=w191, y=T6."Feeding" ("Shooter Mode")) -> (x = y?=w192:bool)
    n116 = Equal?(x=w191, y=T6."Neutral Angle" ("Shooter Mode")) -> (x = y?=w177:bool)
    n117 = Equal?(x=w191, y=T6."Adjust Angle" ("Shooter Mode")) -> (x = y?=w193:bool)
    n118 = Equal?(x=w176, y=WPI_DriverStationRobotMode2."Autonomous Enabled") -> (x = y?=w183:bool)
    n119 = Equal?(x=w176, y=WPI_DriverStationRobotMode2."Teleop Enabled") -> (x = y?=w182:bool)
    n120 = Compound Arithmetic op=OR(w183, w182) -> (w181:bool)
    n121 = Compound Arithmetic op=OR(w193, w192, w177) -> (w188:bool)
    n122 = Compound Arithmetic op=AND(w188, w187, w181) -> (w186:bool)
    n123 = case shown="False" w198 {
      tunnel: [w221 TRUE] -> _
      tunnel: w196 -> [_ w290]
      tunnel: w195 -> [w220 w289]
      tunnel: w194 -> [w219 w291]
      tunnel: w186 -> [w223 _]
      tunnel: w191 -> [w224 _]
      tunnel: w177 -> [w222 _]
      tunnel: w176 -> [w218 _]
      frame False {
        # "Neutral"
        n124 = case shown="True" w223 {
          tunnel: [0.0 ("Numeric") 0.0 ("Numeric")] -> w226
          tunnel: [w238 TRUE] -> w221
          tunnel: w224 -> [w233 _]
          tunnel: w222 -> [_ _]
          tunnel: w220 -> [w231 _]
          tunnel: w219 -> [w230 _]
          tunnel: w218 -> [w229 _]
          frame True {
            # "move Elevator towards target angle"
            n125 = call "Get Target Elevator Angle.vi"("Robot Mode"=w229, "Shooter Mode"=w233) -> ("Target Angle"=w227:dbl)  [unwired: 9 in]
            n126 = In Range and Coerce(upper limit=w231, x=w227, lower limit=w230) -> (coerced(x)=w228:dbl)  [unwired: 1 out]
            n127 = node-c288(i64 10 ("Period")) -> (w237:T7)  [unwired: 2 in]
            n128 = call <vilib>:"SD Write Number.vi"("Numeric"=w228, "Name"="Elevator/Output/Target Angle") -> ()  [unwired: 8 in, 2 out]
            n129 = timed-loop {
              timing: w237 -> [_]
              timing-out: [_] -> w236
              shift-right: [FALSE ("x")] -> _
              shift-left: TRUE ("x") -> [w242]
              tunnel: w233 -> [w253]
              tunnel: [w256] -> w238
              tunnel: w228 -> [w247]
              tunnel: w229 -> [w251]
              stop <- w260 continue-if-true
              # "Same robot/enabled mode"
              # "Same shooter mode"
              # "Angle ready"
              # "re-init if wasn't running"
              # "Target Angle"
              # "Pot Angle"
              n130 = node-c288() -> ()  [unwired: 1 in, 1 out]
              n131 = call "Get Elevator Angle.vi"() -> ("Elevator Angle"=w259:dbl, "Pot Voltage"=w264:dbl)  [unwired: 2 in]
              n132 = local write "Elevator Pot Voltage"(w264) -> ()
              n133 = local write "Elevator Angle"(w259) -> ()
              n134 = global read "Robot Global Data.vi" "UDP Packet"() -> (w244:T12)
              n135 = Unbundle By Name(w244) -> ("Elevator PID Gains"=w243:T3, "Elevator PID Output Range"=w241:cluster{"output high":dbl, "output low":dbl}, "Elevator Angle Tolerance"=w240:dbl)
              n136 = global read "Robot Global Data.vi" "Shooter Mode"() -> (w245:T6)
              n137 = global read "Robot Global Data.vi" "Robot Mode"() -> (w246:T1)
              n138 = Subtract(x=w247, y=w240) -> (x-y=w257:dbl)
              n139 = Add(x=w247, y=w240) -> (x+y=w258:dbl)
              n140 = Equal?(x=w246, y=w251) -> (x = y?=w250:bool)
              n141 = Equal?(x=w245, y=w253) -> (x = y?=w252:bool)
              n142 = In Range and Coerce(upper limit=w258, x=w259, lower limit=w257) -> (In Range?=w256:bool)  [unwired: 1 out]
              n143 = case shown="\"Neutral Angle\"" w253 {
                tunnel: w256 -> [w268 w270 w272 _]
                frame "Adjust Angle" {
                  w267 = FALSE
                  n144 = local write "Shoot Angle Ready"(w268) -> ()
                  n145 = local write "Neutral Angle Ready"(w267) -> ()
                  n146 = local write "Feed Angle Ready"(w267) -> ()
                }
                frame "Feeding" {
                  w269 = FALSE
                  n147 = local write "Feed Angle Ready"(w270) -> ()
                  n148 = local write "Neutral Angle Ready"(w269) -> ()
                  n149 = local write "Shoot Angle Ready"(w269) -> ()
                }
                frame "Neutral Angle" {
                  w271 = FALSE
                  n150 = local write "Neutral Angle Ready"(w272) -> ()
                  n151 = local write "Shoot Angle Ready"(w271) -> ()
                  n152 = local write "Feed Angle Ready"(w271) -> ()
                }
                frame Default {
                }
              }
              n153 = local read "Auto Angle Enabled"() -> (w254:bool)
              n154 = Not(x=w256) -> (.not. x?=w255:bool)
              n155 = call "Get Target Elevator Angle.vi"("Robot Mode"=w246, "Shooter Mode"=w245) -> ("Target Angle"=w248:dbl)  [unwired: 9 in]
              n156 = call-poly <vilib>:"PID.vi"("reinitialize? (F)"=w242, "output range"=w241, "PID gains"=w243, "process variable"=w259, "setpoint"=w247) -> ("output"=w266:dbl)  [unwired: 5 in, 1 out]
              n157 = Equal?(x=w248, y=w247) -> (x = y?=w249:bool)
              n158 = Compound Arithmetic op=AND(w254, w255, w250, w252, w249) -> (w260:bool)
              n159 = Select(t=0.0, s=w256, f=w266) -> (s? t:f=w262:dbl)
              n160 = call "Motor Output Report.vi"("Motor Speed"=w262, "Motor refnum name"="Elevator Motor" ("refnum name")) -> ()  [unwired: 9 in, 1 out]
              n161 = node-c288() -> ()  [unwired: 1 in, 1 out]
            }
            n162 = node-c288(w236) -> ()  [unwired: 1 out]
          }
          frame False {
            # "Elevator not active"
          }
        }
        n163 = call "Motor Output Report.vi"("Motor Speed"=w226, "Motor refnum name"="Elevator Motor" ("refnum name")) -> ()  [unwired: 9 in, 1 out]
      }
      frame True {
        # "Manual"
        # "Within lower limit"
        # "Within upper limit"
        # "Manual override button"
        n164 = global read "Robot Global Data.vi" "Joysticks"() -> (w285:T11)
        n165 = Unbundle By Name(w285) -> ("Manipulator Buttons.Button 10"=w282:bool)
        n166 = global read "Robot Global Data.vi" "Joysticks"() -> (w286:T11)
        n167 = Greater?(x=w289, y=w290) -> (0:w288:bool)
        n168 = Unbundle By Name(w286) -> ("Manipulator Axes.axis 2 (y)"=w296:dbl)
        n169 = Less?(x=w291, y=w290) -> (x < y?=w287:bool)
        n170 = disable-structure shown="Disabled" {
          frame Disabled {
            # "Disable auto elevator"
            n171 = disable-structure shown="Enabled" {
              disable-tunnel: FALSE ("Boolean") -> [w298 w300]
              frame Disabled {
                n172 = call <vilib>:"SD Write Boolean.vi"("Boolean"=w298, "Name"="Elevator/Auto Enabled") -> ()  [unwired: 8 in, 2 out]
              }
              frame Enabled {
                n173 = local write "Elevator Enabled"(w300) -> ()
              }
            }
          }
          frame Enabled {
          }
        }
        n174 = Negate(x=w296) -> (-x=w284:dbl)
        n175 = disable-structure shown="Disabled" {
          disable-tunnel: [w302 TRUE ("Boolean")] -> w294
          frame Disabled {
            n176 = call <vilib>:"SD Read Boolean.vi"("Name"="Motor/Control/Elevator Analog") -> ("Boolean"=w302:bool)  [unwired: 8 in, 2 out]
          }
          frame Enabled {
            # "Elevator Analog"
          }
        }
        n177 = Select(t=w284, s=w282, f=0.0) -> (s? t:f=w283:dbl)
        n178 = call "Joystick Filter.vi"("In"=w283) -> ("Out"=w293:dbl)
        n179 = case shown="True" w294 {
          tunnel: "Elevator Motor" ("refnum name") -> [w312 w320]
          tunnel: w293 -> [w311 w318]
          tunnel: w288 -> [w306 w317]
          tunnel: w287 -> [w305 w319]
          frame False {
            # "Toggle motors"
            n180 = Greater Or Equal?(x=w311, y=0.5) -> (x >= y?=w308:bool)
            n181 = Less Or Equal?(x=w311, y=-0.5) -> (x <= y?=w310:bool)
            n182 = And(x=w305, y=w310) -> (x .and. y?=w309:bool)
            n183 = And(x=w308, y=w306) -> (x .and. y?=w307:bool)
            n184 = call "Motor Output.vi"("Max Power"=1.0, "Backward"=w309, "Forward"=w307, "Motor refnum name"=w312) -> ()  [unwired: 7 in, 1 out]
          }
          frame True {
            # "Joystick to motors"
            n185 = case shown="False" w319 {
              tunnel: w318 -> [w327 w328]
              tunnel: [w325 w328] -> w316
              frame False {
                # "Angle too LOW \nLimit power >0"
                n186 = Max & Min(x=0.0, y=w327) -> (max(x,y)=w325:dbl)  [unwired: 1 out]
              }
              frame True {
                # "Angle not too low"
              }
            }
            n187 = case shown="False" w317 {
              tunnel: w316 -> [w323 w324]
              tunnel: [w321 w324] -> w315
              frame False {
                # "Angle too HIGH\nLimit power <0"
                n188 = Max & Min(x=0.0, y=w323) -> (min(x,y)=w321:dbl)  [unwired: 1 out]
              }
              frame True {
                # "Angle not too high"
              }
            }
            n189 = call "Motor Output Report.vi"("Motor Speed"=w315, "Motor refnum name"=w320) -> ()  [unwired: 9 in, 1 out]
          }
        }
      }
    }
    n190 = call <vilib>:"SD Write Boolean.vi"("Boolean"=w186, "Name"="Elevator/Finding Neutral Angle") -> ()  [unwired: 8 in, 2 out]
  }
  n191 = while {
    stop <- FALSE stop-if-true
    # "Automatic"
    # "Manual"
    n192 = global read "Robot Global Data.vi" "Joysticks"() -> (w333:T11)
    n193 = Unbundle By Name(w333) -> ("Manipulator Buttons.Button 10"=w330:bool, "Manipulator Buttons.Button 11"=w329:bool)
    n194 = case shown="False" w330 {
      tunnel: w329 -> [w334 _]
      frame False {
        n195 = case shown="True" w334 {
          frame False {
          }
          frame True {
            # "Enable auto elevator"
            n196 = local write "Elevator Enabled"(TRUE ("Boolean")) -> ()
          }
        }
      }
      frame True {
        # "Disable auto elevator"
        n197 = local write "Elevator Enabled"(FALSE ("Boolean")) -> ()
      }
    }
    n198 = Wait (ms)(milliseconds to wait=u32 60) -> ()  [unwired: 1 out]
  }
  n199 = while {
    stop <- FALSE stop-if-true
    # "This global is written to in the Autonomous and Teleop VIs"
    # "Flash the USER1 LED with the rate controlled from Autonomous and Teleop"
    n200 = global read "Robot Global Data.vi" "LED toggle rate (ms)"() -> (w337:u32)
    n201 = call <vilib>:"WPI_UtilitiesFRC LEDs.vi"("State"=FPGA_UtilitiesLED_State."Toggle", "LED Type"=FPGA_UtilitiesLED_Source."User LED") -> ()  [unwired: 1 in, 9 out]
    n202 = Wait (ms)(milliseconds to wait=w337) -> ()  [unwired: 1 out]
  }
  n203 = call <vilib>:"WPI_CompressorRefNum Registry Get.vi"("refnum name"="Compressor") -> ("CompressorDevRef"=w25:T21)  [unwired: 9 in, 1 out]
  n204 = call <vilib>:"WPI_CompressorControlLoop.vi"("CompressorDevRef"=w25) -> ()  [unwired: 11 in]
  n205 = call <vilib>:"WPI_DigitalInputRefNum Registry Get.vi"("refnum name"=w2) -> ("DigitalInputDevRef"=w3:T22)  [unwired: 9 in, 1 out]
  n206 = call <vilib>:"WPI_GyroRefNum Registry Get.vi"("refnum name"="Gyro") -> ("GyroDevRef"=w18:T28)  [unwired: 9 in, 1 out]
  n207 = call <vilib>:"WPI_DigitalInputRefNum Registry Get.vi"("refnum name"=w12) -> ("DigitalInputDevRef"=w17:T22)  [unwired: 9 in, 1 out]
  n208 = call <vilib>:"WPI_DigitalInputRefNum Registry Get.vi"("refnum name"=w11) -> ("DigitalInputDevRef"=w16:T22)  [unwired: 9 in, 1 out]
  n209 = call <vilib>:"WPI_DigitalInputRefNum Registry Get.vi"("refnum name"=w4) -> ("DigitalInputDevRef"=w15:T22)  [unwired: 9 in, 1 out]
  n210 = call <vilib>:"WPI_DigitalInputRefNum Registry Get.vi"("refnum name"=w5) -> ("DigitalInputDevRef"=w14:T22)  [unwired: 9 in, 1 out]
  n211 = call <vilib>:"WPI_DigitalInputRefNum Registry Get.vi"("refnum name"=w6) -> ("DigitalInputDevRef"=w13:T22)  [unwired: 9 in, 1 out]
  n212 = call <vilib>:"WPI_EncoderRefNum Registry Get.vi"("refnum name"="Drive Encoder Right") -> ("EncoderDevRef"=w20:T31)  [unwired: 9 in, 1 out]
  n213 = call <vilib>:"WPI_EncoderRefNum Registry Get.vi"("refnum name"="Drive Encoder Left") -> ("EncoderDevRef"=w21:T31)  [unwired: 9 in, 1 out]
  n214 = call <vilib>:"WPI_MotorControlRefNum Registry Get.vi"("refnum name"="Shooter Main") -> ("MotorControlDevRef"=w9:T35)  [unwired: 9 in, 1 out]
  n215 = call <vilib>:"WPI_MotorControlRefNum Registry Get.vi"("refnum name"="Shooter Pre") -> ("MotorControlDevRef"=w7:T35)  [unwired: 9 in, 1 out]
  n216 = while {
    shift-right: [w351] -> _
    shift-left: w21 -> [w364]
    shift-right: [w350] -> _
    shift-left: w20 -> [w400]
    shift-right: [w392] -> _
    shift-left: w18 -> [w397]
    tunnel: w17 -> [w388]
    tunnel: w16 -> [w387]
    tunnel: w15 -> [w386]
    tunnel: w14 -> [w385]
    tunnel: w13 -> [w384]
    tunnel: w12 -> [w383]
    tunnel: w11 -> [w382]
    tunnel: w4 -> [w381]
    tunnel: w5 -> [w380]
    tunnel: w6 -> [w379]
    tunnel: w3 -> [w378]
    tunnel: w2 -> [w377]
    stop <- FALSE stop-if-true
    n217 = disable-structure shown="Disabled" {
      disable-tunnel: [w428 FALSE ("Boolean")] -> w396
      frame Disabled {
        n218 = call <vilib>:"SD Read Boolean.vi"("Name"="Sensor/Gyro/Reset") -> ("Boolean"=w428:bool)  [unwired: 8 in, 2 out]
      }
      frame Enabled {
        # "Reset gryo"
      }
    }
    n219 = disable-structure shown="Disabled" {
      disable-tunnel: w400 -> [w467 w500]
      disable-tunnel: [w466 w496] -> w399
      disable-tunnel: w364 -> [w464 w501]
      disable-tunnel: [w457 w499] -> w351
      disable-tunnel: [w456 w498] -> w350
      frame Disabled {
        n220 = call <vilib>:"SD Read Boolean.vi"("Name"="Encoder/Reset") -> ("Boolean"=w463:bool)  [unwired: 8 in, 2 out]
        n221 = case shown="True" w463 {
          tunnel: w467 -> [w491 w495]
          tunnel: [w491 w494] -> w472
          tunnel: [w490 w493] -> w465
          tunnel: w464 -> [w490 w492]
          frame False {
          }
          frame True {
            n222 = call <vilib>:"WPI_EncoderReset.vi"("EncoderDevRef"=w495) -> ("EncoderDevRef"=w494:T31)  [unwired: 9 in, 1 out]
            n223 = call <vilib>:"WPI_EncoderReset.vi"("EncoderDevRef"=w492) -> ("EncoderDevRef"=w493:T31)  [unwired: 9 in, 1 out]
          }
        }
        n224 = call <vilib>:"SD Read Boolean.vi"("Name"="Encoder/Filter") -> ("Boolean"=w450:bool)  [unwired: 8 in, 2 out]
        n225 = call <vilib>:"WPI_EncoderGet.vi"("EncoderDevRef"=w465) -> ("Distance"=w454:dbl, "EncoderDevRef"=w459:T31, "Rate"=w455:dbl)  [unwired: 5 in, 3 out]
        n226 = call <vilib>:"WPI_EncoderGet.vi"("EncoderDevRef"=w472) -> ("Distance"=w453:dbl, "EncoderDevRef"=w458:T31, "Rate"=w452:dbl)  [unwired: 5 in, 3 out]
        n227 = case shown="True" w450 {
          tunnel: w459 -> [w479 w489]
          tunnel: w458 -> [w476 w488]
          tunnel: [w479 w489] -> w457
          tunnel: [w476 w488] -> w456
          tunnel: w454 -> [w478 w487]
          tunnel: w455 -> [w477 w486]
          tunnel: [w477 w485] -> w449
          tunnel: [w478 w484] -> w432
          tunnel: w452 -> [w474 w483]
          tunnel: w453 -> [w475 w482]
          tunnel: [w475 w481] -> w437
          tunnel: [w474 w480] -> w440
          frame False {
            # "No filtering"
          }
          frame True {
            # "Filter\nEncoders"
            n228 = call-poly <vilib>:"PID Control Input Filter.vi"("input"=w482) -> ("output"=w481:dbl)  [unwired: 4 in]
            n229 = call-poly <vilib>:"PID Control Input Filter.vi"("input"=w483) -> ("output"=w480:dbl)  [unwired: 4 in]
            n230 = call-poly <vilib>:"PID Control Input Filter.vi"("input"=w487) -> ("output"=w484:dbl)  [unwired: 4 in]
            n231 = call-poly <vilib>:"PID Control Input Filter.vi"("input"=w486) -> ("output"=w485:dbl)  [unwired: 4 in]
          }
        }
        n232 = call <vilib>:"SD Read Number.vi"("Name"="Encoder/Right Tick Constant") -> ("Numeric"=w438:dbl)  [unwired: 8 in, 2 out]
        n233 = call <vilib>:"SD Read Number.vi"("Name"="Encoder/Right Constant") -> ("Numeric"=w441:dbl)  [unwired: 8 in, 2 out]
        n234 = call <vilib>:"SD Read Number.vi"("Name"="Encoder/Left Constant") -> ("Numeric"=w444:dbl)  [unwired: 8 in, 2 out]
        n235 = Multiply(x=w437, y=w438) -> (x*y=w433:dbl)
        n236 = Multiply(x=w440, y=w438) -> (x*y=w439:dbl)
        n237 = Multiply(x=w433, y=w441) -> (x*y=w434:dbl)
        n238 = Multiply(x=w439, y=w441) -> (x*y=w448:dbl)
        n239 = Multiply(x=w432, y=w444) -> (x*y=w446:dbl)
        n240 = Multiply(x=w449, y=w444) -> (x*y=w447:dbl)
        n241 = call <vilib>:"SD Write Number.vi"("Numeric"=w448, "Name"="Encoder/Right Speed") -> ()  [unwired: 8 in, 2 out]
        n242 = call <vilib>:"SD Write Number.vi"("Numeric"=w446, "Name"="Encoder/Left Dist") -> ()  [unwired: 8 in, 2 out]
        n243 = call <vilib>:"SD Write Number.vi"("Numeric"=w447, "Name"="Encoder/Left Speed") -> ()  [unwired: 8 in, 2 out]
        n244 = call <vilib>:"SD Write Number.vi"("Numeric"=w434, "Name"="Encoder/Right Dist") -> ()  [unwired: 8 in, 2 out]
        n245 = Add(x=w446, y=w434) -> (x+y=w461:dbl)
        n246 = Divide(x=w461, y=2.0) -> (x/y=w430:dbl)
        n247 = Bundle(cluster=T41 {"Left Dist"=-0.6624599999999999, "Left Speed"=0.0, "Right Dist"=-0.6850325099999999, "Right Speed"=0.0, "Left Ticks"=-91.5, "Right Ticks"=-94.61774999999999, "Avg Distance"=-94.61774999999999, "Avg Speed"=0.0} ("output cluster"), "Left Dist"=w446, "Left Speed"=w447, "Right Dist"=w434, "Right Speed"=w448, "Left Ticks"=w432, "Right Ticks"=w433, "Avg Distance"=w430) -> (w466:T41)  [unwired: 1 in]
        n248 = call <vilib>:"SD Write Number.vi"("Numeric"=w430, "Name"="Encoder/Average Dist") -> ()  [unwired: 8 in, 2 out]
        n249 = call <vilib>:"SD Write Number.vi"("Numeric"=w433, "Name"="Encoder/Right Ticks") -> ()  [unwired: 8 in, 2 out]
        n250 = call <vilib>:"SD Write Number.vi"("Numeric"=w432, "Name"="Encoder/Left Ticks") -> ()  [unwired: 8 in, 2 out]
      }
      frame Enabled {
        n251 = call "Read Encoders.vi"("Reset"=FALSE, "Right Encoder"=w500, "Left Encoder"=w501) -> ("Encoder Values"=w496:T41, "Right Encoder Out"=w498:T31, "Left Encoder Out"=w499:T31)  [unwired: 6 in]
      }
    }
    n252 = call <vilib>:"WPI_DigitalInputGetValue.vi"("DigitalInputDevRef"=w378) -> ("Value"=w376:bool)  [unwired: 8 in, 2 out]
    n253 = call <vilib>:"WPI_DigitalInputGetValue.vi"("DigitalInputDevRef"=w384) -> ("Value"=w373:bool)  [unwired: 8 in, 2 out]
    n254 = call <vilib>:"WPI_DigitalInputGetValue.vi"("DigitalInputDevRef"=w386) -> ("Value"=w370:bool)  [unwired: 8 in, 2 out]
    n255 = call <vilib>:"WPI_DigitalInputGetValue.vi"("DigitalInputDevRef"=w385) -> ("Value"=w372:bool)  [unwired: 8 in, 2 out]
    n256 = call <vilib>:"WPI_DigitalInputGetValue.vi"("DigitalInputDevRef"=w387) -> ("Value"=w368:bool)  [unwired: 8 in, 2 out]
    n257 = call <vilib>:"WPI_DigitalInputGetValue.vi"("DigitalInputDevRef"=w388) -> ("Value"=w366:bool)  [unwired: 8 in, 2 out]
    n258 = Not(x=w370) -> (.not. x?=w369:bool)
    n259 = Not(x=w368) -> (.not. x?=w367:bool)
    n260 = Not(x=w372) -> (.not. x?=w371:bool)
    n261 = Not(x=w366) -> (.not. x?=w365:bool)
    n262 = Not(x=w373) -> (.not. x?=w374:bool)
    n263 = Not(x=w376) -> (.not. x?=w375:bool)
    n264 = First Call?() -> (First Call?: T/F=w389:bool)
    n265 = case shown="False" w389 {
      tunnel: w383 -> [_ w526]
      tunnel: w382 -> [_ w525]
      tunnel: w381 -> [_ w524]
      tunnel: w380 -> [_ w523]
      tunnel: w379 -> [_ w522]
      tunnel: w365 -> [w510 _]
      tunnel: w367 -> [w509 _]
      tunnel: w369 -> [w508 _]
      tunnel: w371 -> [w507 _]
      tunnel: w374 -> [w506 _]
      tunnel: w377 -> [_ w521]
      tunnel: w375 -> [w505 _]
      frame False {
        # "Send DI values all the time"
        n266 = disable-structure shown="Disabled" {
          disable-tunnel: w510 -> [w518 _]
          disable-tunnel: w509 -> [w517 _]
          disable-tunnel: w508 -> [w516 _]
          disable-tunnel: w507 -> [w515 _]
          disable-tunnel: w506 -> [w514 _]
          disable-tunnel: w505 -> [w513 _]
          frame Disabled {
            n267 = Build Array(w518, w517, w516, w515, w514, w513) -> (w520:bool[])
            n268 = call <vilib>:"SD Write Boolean Array.vi"("Boolean Array"=w520, "Name"="Sensor/DI/Values" ("refnum name")) -> ()  [unwired: 8 in, 2 out]
          }
          frame Enabled {
          }
        }
        n269 = global read "Robot Global Data.vi" "IR Sensors"() -> (w512:T42)
        n270 = Bundle By Name(cluster=w512, "Wheel IR 1"=w510, "Wheel IR 2"=w509, "Disc IR Front"=w508, "Disc IR Front 2"=w507, "Disc IR Hopper"=w506, "Disc IR Shooter"=w505) -> (w511:T42)
        n271 = global write "Robot Global Data.vi" "IR Sensors"(w511) -> ()
      }
      frame True {
        # "Send DI names first time only"
        n272 = disable-structure shown="Disabled" {
          disable-tunnel: w526 -> [w532 _]
          disable-tunnel: w525 -> [w531 _]
          disable-tunnel: w524 -> [w530 _]
          disable-tunnel: w523 -> [w529 _]
          disable-tunnel: w522 -> [w528 _]
          disable-tunnel: w521 -> [w527 _]
          frame Disabled {
            n273 = Build Array(w532, w531, w530, w529, w528, w527) -> (w534:string[])
            n274 = call <vilib>:"SD Write String Array.vi"("String Array"=w534, "Name"="Sensor/DI/Names" ("refnum name")) -> ()  [unwired: 8 in, 2 out]
          }
          frame Enabled {
          }
        }
      }
    }
    n275 = case shown="True" w396 {
      tunnel: [w535 w537] -> w398
      tunnel: w397 -> [w535 w536]
      frame False {
      }
      frame True {
        n276 = call <vilib>:"WPI_GyroReset.vi"("GyroDevRef"=w536) -> ("GyroDevRef"=w537:T28)  [unwired: 9 in, 1 out]
      }
    }
    n277 = call <vilib>:"SD Write Number.vi"("Numeric"="Elevator Pot Voltage", "Name"="Sensor/Shooter Pot/Value") -> ()  [unwired: 8 in, 2 out]
    n278 = call <vilib>:"WPI_GyroGetAngle.vi"("GyroDevRef"=w398) -> ("Angular Rate"=w393:dbl, "Angle"=w349:dbl, "GyroDevRef"=w392:T28)  [unwired: 7 in, 1 out]
    n279 = Quotient & Remainder(x=w349, y=360.0) -> (x-y*floor(x/y)=w390:dbl)  [unwired: 1 out]
    n280 = global write "Robot Global Data.vi" "Gryo Angle"(w349) -> ()
    n281 = call <vilib>:"SD Write Number.vi"("Numeric"=w390, "Name"="Sensor/Gyro/Angle") -> ()  [unwired: 8 in, 2 out]
    n282 = call <vilib>:"SD Write Number.vi"("Numeric"=w393, "Name"="Sensor/Gyro/Angular Rate") -> ()  [unwired: 8 in, 2 out]
    n283 = global read "Robot Global Data.vi" "Shooter Mode"() -> (w356:T6)
    n284 = global read "Robot Global Data.vi" "Disc Mode"() -> (w357:enum16{"Drive", "Load", "Shoot", "Feed"})
    n285 = global read "Robot Global Data.vi" "Shoot Location"() -> (w341:T4)
    n286 = local read "Neutral Angle Ready"() -> (w346:bool)
    n287 = disable-structure shown="Enabled" {
      disable-tunnel: "Sensor readings" ("Call Name") -> [w502 w503]
      frame Disabled {
        n288 = call "Loop Delay.vi"("Loop Name"=w502) -> ()  [unwired: 10 in, 1 out]
      }
      frame Enabled {
        n289 = call "Elapsed Times.vi"("Call Name"=w503) -> ()  [unwired: 2 in, 1 out]
        n290 = Wait (ms)(milliseconds to wait=u32 60 ("t")) -> ()  [unwired: 1 out]
      }
    }
    n291 = local read "Shoot Angle Ready"() -> (w352:bool)
    n292 = local read "Feed Angle Ready"() -> (w347:bool)
    n293 = call <vilib>:"SD Write Number.vi"("Numeric"="Elevator Angle", "Name"="Elevator/Angle") -> ()  [unwired: 8 in, 2 out]
    n294 = disable-structure shown="Enabled" {
      disable-tunnel: [w414 w419] -> w358
      disable-tunnel: w357 -> [w413 w420]
      frame Disabled {
        n295 = case shown="\"Shoot\"" w413 {
          tunnel: ["Drive" ("Table Prefix") "Load" ("Table Prefix") "Shoot" ("Table Prefix") "Feed" ("Table Prefix")] -> w414
          frame "Drive", Default {
          }
          frame "Load" {
          }
          frame "Shoot" {
          }
          frame "Feed" {
          }
        }
      }
      frame Enabled {
        n296 = Format Into String(format string="%s", w420) -> (resulting string=w419:string)  [unwired: 2 in, 1 out]
      }
    }
    n297 = disable-structure shown="Enabled" {
      disable-tunnel: w356 -> [w403 w411]
      disable-tunnel: [w402 w410] -> w355
      frame Disabled {
        n298 = case shown="\"Neutral Angle\"" w403 {
          tunnel: ["Wait" ("Table Prefix") "Adjust Angle" ("Table Prefix") "Warmu Shooter" ("Table Prefix") "Fire" ("Table Prefix") "Feeding" ("Table Prefix") "Neutral Angle" ("Table Prefix")] -> w402
          frame "Wait", Default {
          }
          frame "Adjust Angle" {
          }
          frame "Warmup Shooter" {
          }
          frame "Fire" {
          }
          frame "Feeding" {
          }
          frame "Neutral Angle" {
          }
        }
      }
      frame Enabled {
        n299 = Format Into String(format string="%s", w411) -> (resulting string=w410:string)  [unwired: 2 in, 1 out]
      }
    }
    n300 = disable-structure shown="Enabled" {
      disable-tunnel: [w423 w425] -> w343
      disable-tunnel: w341 -> [w422 w426]
      frame Disabled {
        n301 = Flatten To String(anything=w422) -> (data string=w423:string)  [unwired: 3 in, 2 out]
      }
      frame Enabled {
        n302 = Format Into String(format string="%s", w426) -> (resulting string=w425:string)  [unwired: 2 in, 1 out]
      }
    }
    n303 = call <vilib>:"SD Write Boolean.vi"("Boolean"=w352, "Name"="Elevator/Output/Shoot Angle Ready") -> ()  [unwired: 8 in, 2 out]
    n304 = call <vilib>:"SD Write Boolean.vi"("Boolean"=w347, "Name"="Elevator/Output/Feed Angle Ready") -> ()  [unwired: 8 in, 2 out]
    n305 = call <vilib>:"SD Write Boolean.vi"("Boolean"=w346, "Name"="Elevator/Output/Neutral Angle Ready") -> ()  [unwired: 8 in, 2 out]
    n306 = call <vilib>:"SD Write String.vi"("String"=w358, "Name"="Auto/Disc Mode") -> ()  [unwired: 8 in, 2 out]
    n307 = call <vilib>:"SD Write String.vi"("String"=w355, "Name"="Auto/Shooter Mode") -> ()  [unwired: 8 in, 2 out]
    n308 = call <vilib>:"SD Write String.vi"("String"=w343, "Name"="Shoot/Location") -> ()  [unwired: 8 in, 2 out]
    n309 = global write "Robot Global Data.vi" "Encoder Values"(w399) -> ()
  }
  n310 = while {
    tunnel: w9 -> [w546]
    tunnel: w7 -> [w544]
    stop <- FALSE stop-if-true
    # "Send RPM Values"
    n311 = disable-structure shown="Enabled" {
      disable-tunnel: "Shooter Main Loop" ("Call Name") -> [w547 w548]
      frame Disabled {
        n312 = call "Loop Delay.vi"("Loop Name"=w547) -> ()  [unwired: 10 in, 1 out]
      }
      frame Enabled {
        n313 = call "Elapsed Times.vi"("Call Name"=w548) -> ()  [unwired: 2 in, 1 out]
        n314 = Wait (ms)(milliseconds to wait=u32 60 ("t")) -> ()  [unwired: 1 out]
      }
    }
    n315 = call "Get RPM.vi"() -> ("Main RPM"=w539:dbl, "Pre RPM"=w540:dbl)  [unwired: 2 in]
    n316 = global read "Robot Global Data.vi" "Disc Mode"() -> (w543:enum16{"Drive", "Load", "Shoot", "Feed"})
    n317 = local write "Shooter Main RPM"(w539) -> ()
    n318 = local write "Shooter Pre RPM"(w540) -> ()
    n319 = Equal?(x=enum16{"Drive", "Load", "Shoot", "Feed"}."Feed", y=w543) -> (x = y?=w541:bool)
    n320 = case shown="False" w541 {
      tunnel: w546 -> [w552 w629]
      tunnel: w544 -> [w551 w630]
      frame False {
        # "Once in PID/bangbang\nloop, Angle Ready won't be checked"
        n321 = global read "Robot Global Data.vi" "Shooter Active"() -> (w550:bool)
        n322 = case shown="True" w550 {
          tunnel: w552 -> [w554 w558]
          tunnel: w551 -> [w555 w556]
          frame False {
            w553 = 0.0 ("Output")
            n323 = call <vilib>:"WPI_MotorControlSetOutput.vi"("Output"=w553, "MotorControlDevRef"=w555) -> ()  [unwired: 7 in, 3 out]
            n324 = call <vilib>:"WPI_MotorControlSetOutput.vi"("Output"=w553, "MotorControlDevRef"=w554) -> ()  [unwired: 7 in, 3 out]
          }
          frame True {
            n325 = global read "Robot Global Data.vi" "Shooter Manual Power"() -> (w557:bool)
            n326 = case shown="False" w557 {
              tunnel: w558 -> [w561 w620]
              tunnel: w556 -> [w560 w622]
              frame False {
                n327 = disable-structure shown="Disabled" {
                  disable-tunnel: [w562 TRUE ("Boolean")] -> w559
                  frame Disabled {
                    n328 = call <vilib>:"SD Read Boolean.vi"("Name"="Shooter/Bangbang") -> ("Boolean"=w562:bool)  [unwired: 8 in, 2 out]
                  }
                  frame Enabled {
                  }
                }
                n329 = case shown="False" w559 {
                  tunnel: w561 -> [w566 w600]
                  tunnel: w560 -> [w565 w601]
                  frame False {
                    # "PID"
                    n330 = disable-structure shown="Disabled" {
                      disable-tunnel: w566 -> [w568 _]
                      disable-tunnel: w565 -> [w567 _]
                      frame Disabled {
                        n331 = node-c288(i64 10 ("Period")) -> (w572:T7)  [unwired: 2 in]
                        n332 = timed-loop {
                          timing: w572 -> [_]
                          timing-out: [_] -> w571
                          shift-right: [FALSE] -> _
                          shift-left: TRUE -> [w580]
                          shift-right: [w583] -> _
                          shift-left: w567 -> [w587]
                          shift-right: [w581] -> _
                          shift-left: w568 -> [w582]
                          stop <- w590 continue-if-true
                          # "Main"
                          # "Pre"
                          n333 = node-c288() -> ()  [unwired: 1 in, 1 out]
                          n334 = global read "Robot Global Data.vi" "UDP Packet"() -> (w575:T12)
                          n335 = Unbundle By Name(w575) -> ("Shooter PID Gains"=w573:T3, "Shooter PID Output Range"=w574:cluster{"output high":dbl, "output low":dbl})
                          n336 = call "Get RPM.vi"() -> ("Main RPM"=w576:dbl, "Pre RPM"=w577:dbl)  [unwired: 2 in]
                          n337 = local write "Shooter Main RPM"(w576) -> ()
                          n338 = local write "Shooter Pre RPM"(w577) -> ()
                          n339 = global read "Robot Global Data.vi" "Target Main RPM"() -> (w584:dbl)
                          n340 = global read "Robot Global Data.vi" "Target Pre RPM"() -> (w589:dbl)
                          n341 = call-poly <vilib>:"PID.vi"("reinitialize? (F)"=w580, "output range"=w574, "PID gains"=w573, "process variable"=w576, "setpoint"=w584) -> ("output"=w585:dbl)  [unwired: 5 in, 1 out]
                          n342 = call-poly <vilib>:"PID.vi"("reinitialize? (F)"=w580, "output range"=w574, "PID gains"=w573, "process variable"=w577, "setpoint"=w589) -> ("output"=w586:dbl)  [unwired: 5 in, 1 out]
                          n343 = call <vilib>:"WPI_MotorControlSetOutput.vi"("Output"=w585, "MotorControlDevRef"=w582) -> ("Motor Output"=w578:dbl, "MotorControlDevRef"=w581:T35)  [unwired: 7 in, 1 out]
                          n344 = call <vilib>:"WPI_MotorControlSetOutput.vi"("Output"=w586, "MotorControlDevRef"=w587) -> ("Motor Output"=w579:dbl, "MotorControlDevRef"=w583:T35)  [unwired: 7 in, 1 out]
                          n345 = local write "Shooter Main Output"(w578) -> ()
                          n346 = global read "Robot Global Data.vi" "Shooter Active"() -> (w590:bool)
                          n347 = local write "Shooter Pre Output"(w579) -> ()
                          n348 = node-c288() -> ()  [unwired: 1 in, 1 out]
                        }
                        n349 = node-c288(w571) -> ()  [unwired: 1 out]
                      }
                      frame Enabled {
                      }
                    }
                  }
                  frame True {
                    w597 = i64 10 ("Period")
                    # "Bangbang Shooter control"
                    n350 = node-c288(w597) -> (w599:T7)  [unwired: 2 in]
                    n351 = timed-loop {
                      timing: w599 -> [_]
                      timing-out: [_] -> w598
                      tunnel: w601 -> [w612]
                      tunnel: w600 -> [w611]
                      tunnel: w597 -> [w608]
                      stop <- w606 continue-if-true
                      # "Main"
                      # "Pre"
                      n352 = node-c288() -> ()  [unwired: 1 in, 1 out]
                      n353 = global read "Robot Global Data.vi" "Shooter Active"() -> (w606:bool)
                      n354 = call "Get RPM.vi"() -> ("Main RPM"=w602:dbl, "Pre RPM"=w603:dbl)  [unwired: 2 in]
                      n355 = local write "Shooter Main RPM"(w602) -> ()
                      n356 = local write "Shooter Pre RPM"(w603) -> ()
                      n357 = global read "Robot Global Data.vi" "Bangbang Smooth"() -> (w607:dbl)
                      n358 = global read "Robot Global Data.vi" "Target Pre RPM"() -> (w610:dbl)
                      n359 = global read "Robot Global Data.vi" "Target Main RPM"() -> (w609:dbl)
                      n360 = call "Bangbang Shooter Control.vi"("Loop Interval"=w608, "IIR Filter Power"=w607, "Target RPM"=w610, "Current RPM"=w603, "MotorDevRef"=w612) -> ("Motor Output"=w605:dbl)  [unwired: 6 in]
                      n361 = call "Bangbang Shooter Control.vi"("Loop Interval"=w608, "IIR Filter Power"=w607, "Target RPM"=w609, "Current RPM"=w602, "MotorDevRef"=w611) -> ("Motor Output"=w604:dbl)  [unwired: 6 in]
                      n362 = local write "Shooter Pre Output"(w605) -> ()
                      n363 = local write "Shooter Pre Output"(w604) -> ()
                      n364 = node-c288() -> ()  [unwired: 1 in, 1 out]
                    }
                    n365 = node-c288(w598) -> ()  [unwired: 1 out]
                  }
                }
              }
              frame True {
                # "Shoot with powers from dashboard"
                n366 = disable-structure shown="Disabled" {
                  disable-tunnel: [w624 0.5 ("Output")] -> w621
                  disable-tunnel: [w623 0.6 ("Output")] -> w619
                  frame Disabled {
                    n367 = call <vilib>:"SD Read Number.vi"("Name"="Shooter/Shooter Pre" ("refnum name")) -> ("Numeric"=w624:dbl)  [unwired: 8 in, 2 out]
                    n368 = call <vilib>:"SD Read Number.vi"("Name"="Shooter/Shooter Main" ("refnum name")) -> ("Numeric"=w623:dbl)  [unwired: 8 in, 2 out]
                  }
                  frame Enabled {
                  }
                }
                n369 = call <vilib>:"WPI_MotorControlSetOutput.vi"("Output"=w619, "MotorControlDevRef"=w620) -> ()  [unwired: 7 in, 3 out]
                n370 = call <vilib>:"WPI_MotorControlSetOutput.vi"("Output"=w621, "MotorControlDevRef"=w622) -> ()  [unwired: 7 in, 3 out]
                n371 = local write "Shooter Main Output"(w619) -> ()
                n372 = local write "Shooter Pre Output"(w621) -> ()
              }
            }
          }
        }
      }
      frame True {
        n373 = disable-structure shown="Disabled" {
          disable-tunnel: [w634 -0.2 ("Shooter Main Output")] -> w632
          disable-tunnel: [w633 -0.15 ("Shooter Pre Output")] -> w631
          frame Disabled {
            n374 = call <vilib>:"SD Read Number.vi"("Name"="Shooter/Main Feeding" ("refnum name")) -> ("Numeric"=w634:dbl)  [unwired: 8 in, 2 out]
            n375 = call <vilib>:"SD Read Number.vi"("Name"="Shooter/Pre Feeding" ("refnum name")) -> ("Numeric"=w633:dbl)  [unwired: 8 in, 2 out]
          }
          frame Enabled {
          }
        }
        n376 = local write "Shooter Pre Output"(w631) -> ()
        n377 = local write "Shooter Main Output"(w632) -> ()
        n378 = call <vilib>:"WPI_MotorControlSetOutput.vi"("Output"=w632, "MotorControlDevRef"=w629) -> ()  [unwired: 7 in, 3 out]
        n379 = call <vilib>:"WPI_MotorControlSetOutput.vi"("Output"=w631, "MotorControlDevRef"=w630) -> ()  [unwired: 7 in, 3 out]
      }
    }
  }
  n380 = while {
    stop <- FALSE stop-if-true
    # "Solenoid\n\nF - 1st gear\nT - 2nd gear"
    # "Flipper"
    # "Hopper"
    # "Auto Loading"
    # "Auto Loading"
    # "Location selected"
    # "Shoot case"
    # "Shoot Button"
    # "Manual Buttons"
    # "Assume Disc count is bad"
    # "Find Neutral Angle when Disabled"
    # "Enabled?"
    # "Exit all modes when Disabled"
    # "Elevator active in:\n     Adjust Angle\n     Feeding\n     Wait (neutral angle)"
    # "Reverse Right roller"
    # "Rollers forward"
    # "Rollers backward"
    # "Same as Left, unless 2 Disc detected"
    # "Take commands direct from Auto logic"
    # "Intercept Auto Right roller\ncommands, force reverse if 2 discs"
    # "Bck"
    # "Fwd"
    # "Bck"
    # "Fwd"
    # "Reverse Right roller"
    # "Manual Load"
    # "Both IRs"
    # "1+ IR"
    # "Elevator/Auto Enabled"
    # "NOTE: Manual shooter power keeps\nshooter in Warmup mode (user fires manually)"
    # "Shooter Mode:\n Wait - nothing\n Adjust Angle - run elevator\n Warmup Shooter - run shoot loop (PID/manual)\n Fire - deploy Flipper"
    # "Rollers backward"
    # "Rollers forward"
    # "Flipper piston (direct from solenoid)"
    # "Manual control => loader ramp down"
    # "Hopper full"
    # "Loading"
    # "Rollers moving?"
    # "Flipper"
    # "Hopper"
    # "Lower Loader Ramp and Hopper"
    # "last Disc Mode"
    # "Feed"
    n381 = disable-structure shown="Disabled" {
      frame Disabled {
        (unwired) WPI_DriverStationRobotMode2."Teleop Enabled" ("x")
        n382 = global read "Robot Global Data.vi" "Robot Mode"() -> (w857:T1)
        n383 = Equal?(x=w857) -> (x = y?=w854:bool)  [unwired: 1 in]
        n384 = feedback #1() -> (w856:T1)  [unwired: 1 in]
        n385 = Not Equal?(x=w856, y=w857) -> (x != y?=w855:bool)
        n386 = feedback-in #1(w857) -> ()
        n387 = And(x=w855, y=w854) -> ()  [unwired: 1 out]
      }
      frame Enabled {
      }
    }
    n388 = global read "Robot Global Data.vi" "Auton Commands"() -> (w752:T5)
    n389 = global read "Robot Global Data.vi" "Joysticks"() -> (w699:T11)
    n390 = global read "Robot Global Data.vi" "Joysticks"() -> (w700:T11)
    n391 = Unbundle By Name(w699) -> ("Driver Buttons"=w698:T10)
    n392 = Unbundle By Name(w700) -> ("Manipulator Buttons"=w701:T10)
    n393 = global read "Robot Global Data.vi" "IR Sensors"() -> (w826:T42)
    n394 = disable-structure shown="Enabled" {
      disable-tunnel: [w876 TRUE] -> w718
      frame Disabled {
        n395 = global read "Robot Global Data.vi" "Halo Drive"() -> (w876)
      }
      frame Enabled {
        # "Halo?"
      }
    }
    n396 = global read "Robot Global Data.vi" "Robot Mode"() -> (w822:T1)
    n397 = disable-structure shown="Enabled" {
      disable-tunnel: "Auto Logic" ("Call Name") -> [w885 w886]
      frame Disabled {
        n398 = call "Loop Delay.vi"("Loop Name"=w885) -> ()  [unwired: 10 in, 1 out]
      }
      frame Enabled {
        n399 = call "Elapsed Times.vi"("Call Name"=w886) -> ()  [unwired: 2 in, 1 out]
        n400 = Wait (ms)(milliseconds to wait=u32 40 ("t")) -> ()  [unwired: 1 out]
      }
    }
    n401 = global read "Robot Global Data.vi" "Robot Mode"() -> (w739:T1)
    n402 = Unbundle By Name(w752) -> ("Warmup"=w642:bool, "Shoot"=w751:bool)
    n403 = Unbundle By Name(w701) -> ("Button 2"=w820:bool, "Button 3"=w827:bool)
    n404 = Unbundle By Name(w826) -> ("Disc IR Front"=w763:bool, "Disc IR Front 2"=w764:bool)
    n405 = global read "Robot Global Data.vi" "Target Pre RPM"() -> (w807:dbl)
    n406 = case shown="False" w718 {
      tunnel: [w1119 w1121] -> w724
      tunnel: w698 -> [w1118 w1120]
      frame False {
        # "Joystick"
        n407 = Unbundle By Name(w1118) -> ("Button 2"=w1119:bool)
      }
      frame True {
        # "Gamepad"
        n408 = Unbundle By Name(w1120) -> ("Button 6"=w1121:bool)
      }
    }
    n409 = global read "Robot Global Data.vi" "Target Main RPM"() -> (w811:dbl)
    n410 = Equal?(x=WPI_DriverStationRobotMode2."Autonomous Enabled", y=w822) -> (x = y?=w641:bool)
    n411 = global read "Robot Global Data.vi" "RPM Min Percentage"() -> (w812:dbl)
    n412 = global read "Robot Global Data.vi" "Robot Mode"() -> (w750:T1)
    n413 = global read "Robot Global Data.vi" "Joysticks"() -> (w691:T11)
    n414 = Unbundle By Name(w691) -> ("Manipulator Axes"=w690:T43, "Manipulator Buttons"=w689:T10)
    n415 = Equal?(x=w739, y=WPI_DriverStationRobotMode2."Teleop Enabled" ("x")) -> (x = y?=w737:bool)
    n416 = Equal?(x=w739, y=WPI_DriverStationRobotMode2."Autonomous Enabled" ("x")) -> (x = y?=w736:bool)
    n417 = disable-structure shown="Enabled" {
      disable-tunnel: [w883 0.0 ("Disc Count")] -> w770
      frame Disabled {
        n418 = global read "Robot Global Data.vi" "Disc Count"() -> (w883:dbl)
      }
      frame Enabled {
      }
    }
    n419 = global read "Robot Global Data.vi" "RPM Max Percentage"() -> (w813:dbl)
    n420 = Compound Arithmetic op=OR(w736, w737) -> (w730:bool)
    n421 = Select(t=w751, s=w641, f=w820) -> (s? t:f=w643:bool)
    n422 = And(x=w641, y=w642) -> (x .and. y?=w640:bool)
    n423 = Equal?(x=WPI_DriverStationRobotMode2."Autonomous Enabled", y=w750) -> (x = y?=w726:bool)
    n424 = Or(x=w763, y=w764) -> (x .or. y?=w819:bool)
    n425 = And(x=w763, y=w764) -> (x .and. y?=w723:bool)
    n426 = Multiply(x=w812, y=w807) -> (x*y=w809:dbl)
    n427 = Multiply(x=w812, y=w811) -> (x*y=w815:dbl)
    n428 = disable-structure shown="Enabled" {
      disable-tunnel: [w869 FALSE ("Boolean")] -> w762
      frame Disabled {
        n429 = call <vilib>:"SD Read Boolean.vi"("Name"="Auto/Loading Enabled") -> ("Boolean"=w869:bool)  [unwired: 8 in, 2 out]
      }
      frame Enabled {
      }
    }
    n430 = call "Get Manipulator Shoot Location.vi"("Manipulator Buttons"=w689, "Manipulator Axes"=w690) -> ("Manual Buttons"=w665:T44, "Shoot Location"=w688:T4, "Location Selected"=w644:bool)  [unwired: 7 in]
    n431 = And(x=w819, y=w762) -> (x .and. y?=w722:bool)
    n432 = And(x=w762, y=w723) -> (x .and. y?=w720:bool)
    n433 = case shown="True" w726 {
      tunnel: [w879 w881] -> w721
      tunnel: [w878 w880] -> w725
      tunnel: w720 -> [w879 _]
      tunnel: w724 -> [w878 _]
      frame False {
        # "Teleop"
        # "Both IRs"
        # "Manual Load"
      }
      frame True {
        # "Autonomous"
        n434 = global read "Robot Global Data.vi" "Auton Commands"() -> (w882:T5)
        n435 = Unbundle By Name(w882) -> ("Two Discs"=w881:bool, "Load"=w880:bool)
      }
    }
    n436 = Multiply(x=w813, y=w807) -> (x*y=w808:dbl)
    n437 = global read "Robot Global Data.vi" "Shooter Mode"() -> (w733:T6)
    n438 = feedback #2() -> (w741:enum16{"Drive", "Load", "Shoot", "Feed"})  [unwired: 1 in]
    n439 = local read "Shooter Pre RPM"() -> (w810:dbl)
    n440 = Multiply(x=w813, y=w811) -> (x*y=w814:dbl)
    n441 = global read "Robot Global Data.vi" "Disc Mode"() -> (w735:enum16{"Drive", "Load", "Shoot", "Feed"})
    n442 = local read "Shooter Main RPM"() -> (w816:dbl)
    n443 = global read "Robot Global Data.vi" "UDP Packet"() -> (w710:T12)
    n444 = global write "Robot Global Data.vi" "Shoot Location"(w688) -> ()
    n445 = Compound Arithmetic op=OR(w640, w643, w644) -> (w645:bool)
    n446 = feedback-in #3(w688) -> ()
    n447 = feedback #3() -> (w687:T4)  [unwired: 1 in]
    n448 = Select(t=w735, s=w730, f=enum16{"Drive", "Load", "Shoot", "Feed"}."Drive") -> (s? t:f=w693:enum16{"Drive", "Load", "Shoot", "Feed"})
    n449 = feedback-in #2(w693) -> ()
    n450 = Select(t=w733, s=w730, f=T6."Neutral Angle") -> (s? t:f=w731:T6)
    n451 = Greater Or Equal?(x=w770, y=4.0) -> (x >= y?=w786:bool)
    n452 = case shown="\"Shoot\"" w693 {
      selector: w693 -> [w914 w958 w1029 w1102]
      tunnel: w645 -> [w916 w967 w1004 _]
      tunnel: [w917 w965 w1028 w1101] -> w666
      tunnel: w827 -> [w915 w962 _ w1100]
      tunnel: [FALSE ("Drive Limit") TRUE ("Drive Limit") FALSE ("Drive Limit") FALSE ("Drive Limit")] -> w683
      tunnel: w770 -> [_ _ w1020 _]
      tunnel: [FALSE FALSE TRUE FALSE] -> w791
      tunnel: [w892 w923 w1018 w1095] -> w648
      tunnel: [w905 w947 w1023 w1097] -> w757
      tunnel: w741 -> [_ w952 w1017 _]
      tunnel: [w905 w948 w1023 w1097] -> w790
      tunnel: w722 -> [w911 w943 _ _]
      tunnel: w786 -> [w907 w945 _ _]
      tunnel: w725 -> [w910 w926 _ _]
      tunnel: [w900 w934 w1003 T6."Feeding" ("Shooter Mode")] -> w685
      tunnel: w721 -> [_ w940 _ _]
      tunnel: [w905 w939 w1023 w1097] -> w760
      tunnel: w731 -> [w903 w935 _ _]
      tunnel: w710 -> [_ _ w1010 _]
      tunnel: w688 -> [_ _ w1001 _]
      tunnel: w643 -> [_ _ w997 _]
      tunnel: w687 -> [_ _ w1002 _]
      tunnel: [w892 w923 w997 w1095] -> w646
      frame "Drive", Default {
        w905 = FALSE ("Elevator Active")
        w892 = FALSE
        # "activate Neutral Angle, then wait"
        n453 = local read "Elevator Neutral Enabled"() -> (w893:bool)
        n454 = local read "Auto Angle Enabled"() -> (w899:bool)
        n455 = Or(x=w911, y=w910) -> (x .or. y?=w909:bool)
        n456 = local read "Neutral Angle Ready"() -> (w896:bool)
        n457 = Not(x=w899) -> (.not. x?=w895:bool)
        n458 = Equal?(x=w903, y=T6."Wait" ("Shooter Mode")) -> (x = y?=w897:bool)
        n459 = Not(x=w893) -> (.not. x?=w894:bool)
        n460 = Compound Arithmetic op=OR(w895, w896, w897, w894) -> (w898:bool)
        n461 = Not(x=w907) -> (.not. x?=w908:bool)
        n462 = And(x=w908, y=w909) -> (x .and. y?=w906:bool)
        n463 = Select(t=T6."Wait" ("Shooter Mode"), s=w898, f=T6."Neutral Angle" ("Shooter Mode")) -> (s? t:f=w900:T6)
        n464 = Select(t=enum16{"Drive", "Load", "Shoot", "Feed"}."Load", s=w906, f=w914) -> (s? t:f=w919:enum16{"Drive", "Load", "Shoot", "Feed"})
        n465 = Select(t=enum16{"Drive", "Load", "Shoot", "Feed"}."Feed", s=w915, f=w919) -> (s? t:f=w918:enum16{"Drive", "Load", "Shoot", "Feed"})
        n466 = Select(t=enum16{"Drive", "Load", "Shoot", "Feed"}."Shoot", s=w916, f=w918) -> (s? t:f=w917:enum16{"Drive", "Load", "Shoot", "Feed"})
      }
      frame "Load" {
        w923 = FALSE
        # "activate Neutral Angle, then wait"
        # "Both IRs?"
        # "stop if hopper full, or no discs found"
        # "Loading start time"
        # "Was Loading?"
        # "TODO"
        # "TODO: pick up multiple discs, stop when\nthe last disc crosses the Hopper IR"
        n467 = disable-structure shown="Disabled" {
          disable-tunnel: [w976 "Load Exit Delay (ms)"] -> w955
          frame Disabled {
            n468 = call <vilib>:"SD Read Number.vi"("Name"="Auto/Load Exit Delay") -> ("Numeric"=w976:dbl)  [unwired: 8 in, 2 out]
          }
          frame Enabled {
          }
        }
        n469 = disable-structure shown="Enabled" {
          disable-tunnel: [w973 "Load Roller Delay (ms)"] -> w949
          frame Disabled {
            n470 = call <vilib>:"SD Read Number.vi"("Name"="Auto/Load Roller Delay") -> ("Numeric"=w973:dbl)  [unwired: 8 in, 2 out]
          }
          frame Enabled {
          }
        }
        n471 = local read "Auto Angle Enabled"() -> (w929:bool)
        n472 = local read "Elevator Neutral Enabled"() -> (w927:bool)
        n473 = Not(x=w945) -> (.not. x?=w944:bool)
        n474 = local read "Neutral Angle Ready"() -> (w930:bool)
        n475 = And(x=w944, y=w943) -> (x .and. y?=w924:bool)
        n476 = Or(x=w924, y=w926) -> (x .or. y?=w925:bool)
        n477 = Equal?(x=enum16{"Drive", "Load", "Shoot", "Feed"}."Load" ("f"), y=w952) -> (x = y?=w954:bool)
        n478 = Not(x=w929) -> (.not. x?=w933:bool)
        n479 = Equal?(x=w935, y=T6."Wait" ("Shooter Mode")) -> (x = y?=w931:bool)
        n480 = disable-structure shown="Disabled" {
          disable-tunnel: [w969 "Two Disc Loading"] -> w941
          frame Disabled {
            n481 = call <vilib>:"SD Read Boolean.vi"("Name"="Auto/Two Disc Loading") -> ("Boolean"=w969:bool)  [unwired: 8 in, 2 out]
          }
          frame Enabled {
          }
        }
        n482 = Not(x=w927) -> (.not. x?=w928:bool)
        n483 = feedback #4() -> (w956:u32)  [unwired: 1 in]
        n484 = case shown="True" w925 {
          tunnel: [w993 w996] -> w957
          tunnel: w956 -> [w993 _]
          tunnel: [w991 FALSE] -> w942
          tunnel: w955 -> [w990 _]
          frame False {
            # "No disc in last X seconds"
            n485 = Tick Count (ms)() -> (millisecond timer value=w994:u32)
            n486 = Subtract(x=w994, y=w993) -> (x-y=w992:u32)
            n487 = Greater?(x=w992, y=w990) -> (0:w991:bool)
          }
          frame True {
            n488 = Tick Count (ms)() -> (millisecond timer value=w996:u32)
          }
        }
        n489 = disable-structure shown="Enabled" {
          disable-tunnel: [w979 w981] -> w946
          disable-tunnel: w942 -> [w978 w981]
          frame Disabled {
            # "only exit if NOT manual"
            n490 = Not() -> (.not. x?=w980:bool)  [unwired: 1 in]
            n491 = And(x=w980, y=w978) -> (x .and. y?=w979:bool)
          }
          frame Enabled {
          }
        }
        n492 = feedback-in #4(w957) -> ()
        n493 = Compound Arithmetic op=OR(w933, w930, w931, w928) -> (w932:bool)
        n494 = Select(t=T6."Wait" ("Shooter Mode"), s=w932, f=T6."Neutral Angle" ("Shooter Mode")) -> (s? t:f=w934:T6)
        n495 = And(x=w941, y=w940) -> (x .and. y?=w939:bool)
        n496 = Select(t=enum16{"Drive", "Load", "Shoot", "Feed"}."Drive", s=w946, f=w958) -> (s? t:f=w963:enum16{"Drive", "Load", "Shoot", "Feed"})
        n497 = feedback #5() -> (w950:u32)  [unwired: 1 in]
        n498 = case shown="True" w954 {
          tunnel: [w983 w984] -> w951
          tunnel: w950 -> [_ w984]
          tunnel: w949 -> [_ w987]
          tunnel: [w982 w986] -> w948
          tunnel: [w982 w985] -> w947
          frame False {
            w982 = FALSE
            # "First time in Load case, record\nLoad start time"
            n499 = Tick Count (ms)() -> (millisecond timer value=w983:u32)
          }
          frame True {
            # "Delay finished"
            # "If delay time has elapsed,\nrun the rollers"
            n500 = Tick Count (ms)() -> (millisecond timer value=w989:u32)
            n501 = Subtract(x=w989, y=w984) -> (x-y=w988:u32)
            n502 = Greater Or Equal?(x=w988, y=w987) -> (x >= y?=w985:bool)
            n503 = Not(x=w985) -> (.not. x?=w986:bool)
          }
        }
        n504 = feedback-in #5(w951) -> ()
        n505 = Select(t=enum16{"Drive", "Load", "Shoot", "Feed"}."Feed", s=w962, f=w963) -> (s? t:f=w961:enum16{"Drive", "Load", "Shoot", "Feed"})
        n506 = Select(t=enum16{"Drive", "Load", "Shoot", "Feed"}."Shoot", s=w967, f=w961) -> (s? t:f=w965:enum16{"Drive", "Load", "Shoot", "Feed"})
      }
      frame "Shoot" {
        w1023 = FALSE ("Elevator Active")
        # "if not shooter button, only Adjust Angle"
        # "exit Shoot?"
        # "Discs or Manual"
        # "Hopper has discs"
        n507 = local read "Auto Angle Enabled"() -> (w1013:bool)
        n508 = Greater Than 0?(x=w1020) -> (x > 0?=w1022:bool)
        n509 = Not Equal?(x=enum16{"Drive", "Load", "Shoot", "Feed"}."Shoot", y=w1017) -> (x != y?=w999:bool)
        n510 = Not Equal?(x=w1001, y=w1002) -> (x != y?=w998:bool)
        n511 = local read "RPM Ready"() -> (w1012:bool)
        n512 = global read "Robot Global Data.vi" "Shooter Mode"() -> (w1024:T6)
        n513 = Or(x=w1004, y=w1022) -> (x .or. y?=w1021:bool)
        n514 = Compound Arithmetic op=OR(w999, w998) -> (w1000:bool)
        n515 = feedback #6() -> (w1025:u32)  [unwired: 1 in]
        n516 = case shown="False" w1021 {
          tunnel: [w1088 w1094] -> w1026
          tunnel: w1025 -> [w1088 _]
          tunnel: [w1086 FALSE] -> w1019
          frame False {
            # "elapsed time"
            # "No disc in last 0.5 seconds"
            n517 = Tick Count (ms)() -> (millisecond timer value=w1089:u32)
            n518 = Subtract(x=w1089, y=w1088) -> (x-y=w1087:u32)
            n519 = disable-structure shown="Disabled" {
              disable-tunnel: [w1090 "Shoot Exit Delay (ms)"] -> w1085
              frame Disabled {
                n520 = call <vilib>:"SD Read Number.vi"("Name"="Auto/Shoot Exit Delay") -> ("Numeric"=w1090:dbl)  [unwired: 8 in, 2 out]
              }
              frame Enabled {
              }
            }
            n521 = Greater?(x=w1087, y=w1085) -> (0:w1086:bool)
          }
          frame True {
            # "Record time user wanted to shoot"
            n522 = Tick Count (ms)() -> (millisecond timer value=w1094:u32)
          }
        }
        n523 = feedback-in #6(w1026) -> ()
        n524 = case shown="\"Fire\"" w1024 {
          selector: w1024 -> [_ w1063 w1074 w1084]
          tunnel: w1013 -> [w1059 w1066 _ _]
          tunnel: [w1058 w1064 w1075 w1083] -> w1003
          tunnel: w1012 -> [_ _ w1072 w1079]
          tunnel: w997 -> [_ _ w1067 w1076]
          frame "Wait", "Feeding", "Neutral Angle", Default {
            # "Skip to warmup if auto angle disabled"
            n525 = Select(t=T6."Adjust Angle" ("Shooter Mode"), s=w1059, f=T6."Warmup Shooter" ("Shooter Mode")) -> (s? t:f=w1058:T6)
          }
          frame "Adjust Angle" {
            # "Skip to warmup if angle ready,\nor if auto angle disabled"
            n526 = local read "Shoot Angle Ready"() -> (w1061:bool)
            n527 = Not(x=w1066) -> (.not. x?=w1062:bool)
            n528 = Or(x=w1062, y=w1061) -> (x .or. y?=w1065:bool)
            n529 = Select(t=T6."Warmup Shooter" ("Shooter Mode"), s=w1065, f=w1063) -> (s? t:f=w1064:T6)
          }
          frame "Warmup Shooter" {
            # "If not manual and\nRPM and Azimuth \nready, fire"
            n530 = global read "Robot Global Data.vi" "Shooter Manual Power"() -> (w1073:bool)
            n531 = global read "Robot Global Data.vi" "Azimuth Ready"() -> (w1069:bool)
            n532 = Not(x=w1073) -> (.not. x?=w1071:bool)
            n533 = Compound Arithmetic op=AND(w1071, w1072, w1069, w1067) -> (w1070:bool)
            n534 = Select(t=T6."Fire" ("Shooter Mode"), s=w1070, f=w1074) -> (s? t:f=w1075:T6)
          }
          frame "Fire" {
            # "If not manual or RPM and Azimuth\n ready, fire otherwise, warmup"
            n535 = global read "Robot Global Data.vi" "Shooter Manual Power"() -> (w1082:bool)
            n536 = global read "Robot Global Data.vi" "Azimuth Ready"() -> (w1078:bool)
            n537 = Not(x=w1082) -> (.not. x?=w1081:bool)
            n538 = Compound Arithmetic op=AND(w1081, w1079, w1078, w1076) -> (w1080:bool)
            n539 = Select(t=w1084, s=w1080, f=T6."Warmup Shooter" ("Shooter Mode")) -> (s? t:f=w1083:T6)
          }
        }
        n540 = feedback #7() -> (w1009:T15)  [unwired: 1 in]
        n541 = case shown="True" w1000 {
          tunnel: w1001 -> [_ w1033]
          tunnel: w1010 -> [_ w1032]
          tunnel: [w1030 w1031] -> w1008
          tunnel: w1009 -> [w1030 _]
          frame False {
            # "Keep same distance and\nRPM while shooting"
          }
          frame True {
            # "Grab distance and RPM\nwhen shooting starts"
            n542 = case shown="\"Back Corner\"" w1033 {
              tunnel: w1032 -> [w1035 w1037 w1039 w1041 w1043 w1045 w1047]
              tunnel: [w1034 w1036 w1038 w1040 w1042 w1044 w1046] -> w1031
              frame "Vision", Default {
                n543 = Unbundle By Name(w1035) -> ("Shoot Setpoints.Vision"=w1034:T15)
              }
              frame "Front" {
                n544 = Unbundle By Name(w1037) -> ("Shoot Setpoints.Front"=w1036:T15)
              }
              frame "Front Corner" {
                n545 = Unbundle By Name(w1039) -> ("Shoot Setpoints.Front Corner"=w1038:T15)
              }
              frame "Back Corner" {
                n546 = Unbundle By Name(w1041) -> ("Shoot Setpoints.Back Corner"=w1040:T15)
              }
              frame "Half Court" {
                n547 = Unbundle By Name(w1043) -> ("Shoot Setpoints.Half Court"=w1042:T15)
              }
              frame "Full Court" {
                n548 = Unbundle By Name(w1045) -> ("Shoot Setpoints.Full Court"=w1044:T15)
              }
              frame "Pyramid" {
                n549 = Unbundle By Name(w1047) -> ("Shoot Setpoints.Pyramid"=w1046:T15)
              }
            }
          }
        }
        n550 = feedback-in #7(w1008) -> ()
        n551 = disable-structure shown="Enabled" {
          disable-tunnel: w1029 -> [w1051 w1054]
          disable-tunnel: [w1049 w1055] -> w1028
          disable-tunnel: w1004 -> [w1048 _]
          disable-tunnel: w1019 -> [_ w1052]
          frame Disabled {
            n552 = Select(t=w1051, s=w1048, f=enum16{"Drive", "Load", "Shoot", "Feed"}."Drive") -> (s? t:f=w1049:enum16{"Drive", "Load", "Shoot", "Feed"})
          }
          frame Enabled {
            n553 = Select(t=enum16{"Drive", "Load", "Shoot", "Feed"}."Drive" ("f"), s=w1052, f=w1054) -> (s? t:f=w1055:enum16{"Drive", "Load", "Shoot", "Feed"})
          }
        }
        n554 = Unbundle By Name(w1008) -> ("Pre RPM"=w1007:dbl, "Main RPM"=w1006:dbl, "Angle"=w1005:dbl)
        n555 = global write "Robot Global Data.vi" "Elevator Target Angle"(w1005) -> ()
        n556 = global write "Robot Global Data.vi" "Target Main RPM"(w1006) -> ()
        n557 = global write "Robot Global Data.vi" "Target Pre RPM"(w1007) -> ()
        n558 = Equal?(x=w1003, y=T6."Fire" ("Shooter Mode")) -> (x = y?=w1011:bool)
        n559 = And(x=w997, y=w1011) -> (x .and. y?=w1018:bool)
      }
      frame "Feed" {
        w1097 = FALSE ("Elevator Active")
        w1095 = FALSE
        # "When feeding, hopper is down"
        n560 = Select(t=w1102, s=w1100, f=enum16{"Drive", "Load", "Shoot", "Feed"}."Drive") -> (s? t:f=w1101:enum16{"Drive", "Load", "Shoot", "Feed"})
      }
    }
    n561 = In Range and Coerce(upper limit=w808, x=w810, lower limit=w809) -> (In Range?=w805:bool)  [unwired: 1 out]
    n562 = In Range and Coerce(upper limit=w814, x=w816, lower limit=w815) -> (In Range?=w806:bool)  [unwired: 1 out]
    n563 = And(x=w805, y=w806) -> (x .and. y?=w765:bool)
    "RPM Ready" <- w765
    n564 = call <vilib>:"SD Write Boolean.vi"("Boolean"=w765, "Name"="Shooter/Output/RPM Ready") -> ()  [unwired: 8 in, 2 out]
    n565 = disable-structure shown="Enabled" {
      disable-tunnel: [w865 w868] -> w768
      disable-tunnel: [w861 w868] -> w767
      disable-tunnel: [w860 w868] -> w766
      frame Disabled {
        # "D-pad left (subtract 1)"
        # "D-pad right (add 1)"
        # "D-pad up (reset count)"
        n566 = global read "Robot Global Data.vi" "Joysticks"() -> (w859:T11)
        n567 = Unbundle By Name(w859) -> ("Manipulator Axes"=w858:T43)
        n568 = Unbundle By Name(w858) -> ("axis 5"=w862:dbl, "axis 6"=w867:dbl)
        n569 = Less?(x=w867, y=-0.5) -> (x < y?=w865:bool)
        n570 = Greater?(x=w862, y=0.5) -> (0:w861:bool)
        n571 = Less?(x=w862, y=-0.5) -> (x < y?=w860:bool)
      }
      frame Enabled {
        w868 = FALSE ("Manual Add")
        # "No disc mode manual\ncontrol, not used"
      }
    }
    n572 = call <vilib>:"SD Write Boolean.vi"("Boolean"=w648, "Name"="Shooter/Output/Flipper Output") -> ()  [unwired: 8 in, 2 out]
    n573 = global write "Robot Global Data.vi" "Shooter Mode"(w685) -> ()
    n574 = global write "Robot Global Data.vi" "Disc Mode"(w666) -> ()
    n575 = global read "Robot Global Data.vi" "Joysticks"() -> (w697:T11)
    n576 = Unbundle By Name(w697) -> ("Manipulator Buttons"=w696:T10)
    n577 = global read "Robot Global Data.vi" "IR Sensors"() -> (w769:T42)
    n578 = Equal?(x=w685, y=T6."Adjust Angle" ("Shooter Mode")) -> (x = y?=w684:bool)
    n579 = Equal?(x=w685, y=T6."Fire" ("Shooter Mode")) -> (x = y?=w714:bool)
    n580 = Equal?(x=w685, y=T6."Warmup Shooter" ("Shooter Mode")) -> (x = y?=w713:bool)
    n581 = Compound Arithmetic op=OR(w684, w713, w714) -> (w712:bool)
    n582 = call <vilib>:"SD Write Boolean.vi"("Boolean"=w712, "Name"="Shooter/Output/Shooter Ready") -> ()  [unwired: 8 in, 2 out]
    n583 = global write "Robot Global Data.vi" "Shooter Active"(w712) -> ()
    n584 = Unbundle By Name(w696) -> ("Button 1"=w651:bool, "Button 5"=w782:bool, "Button 7"=w778:bool, "Button 6"=w780:bool, "Button 8"=w777:bool)
    n585 = disable-structure shown="Disabled" {
      disable-tunnel: [w872 "Load Reverse Enabled"] -> w761
      frame Disabled {
        n586 = call <vilib>:"SD Read Boolean.vi"("Name"="Auto/Load Reverse Enabled") -> ("Boolean"=w872:bool)  [unwired: 8 in, 2 out]
      }
      frame Enabled {
      }
    }
    n587 = disable-structure shown="Enabled" {
      disable-tunnel: [_ TRUE] -> w717
      frame Disabled {
        # "Halo?"
        n588 = global read "Robot Global Data.vi" "Halo Drive"() -> ()  [unwired: 1 out]
      }
      frame Enabled {
        # "Halo?"
      }
    }
    n589 = Unbundle By Name(w769) -> ("Disc IR Shooter"=w824:bool, "Disc IR Hopper"=w825:bool)
    n590 = global read "Robot Global Data.vi" "Joysticks"() -> (w695:T11)
    n591 = Unbundle By Name(w695) -> ("Driver Buttons"=w694:T10)
    n592 = disable-structure shown="Enabled" {
      disable-tunnel: w651 -> [w850 w853]
      disable-tunnel: [w849 w851] -> w792
      disable-tunnel: w791 -> [w847 w852]
      frame Disabled {
        n593 = call "Button Toggle.vi"("Button Input"=w850) -> ("Toggled Output"=w848:bool)  [unwired: 4 in]
        n594 = Or(x=w848, y=w847) -> (x .or. y?=w849:bool)
      }
      frame Enabled {
        n595 = Exclusive Or(1:w852, 2:w853) -> (0:w851:bool)
      }
    }
    n596 = global read "Robot Global Data.vi" "Disc Mode"() -> (w692:enum16{"Drive", "Load", "Shoot", "Feed"})
    n597 = Compound Arithmetic op=OR(w782, w778, w780, w777) -> (w682:bool)
    n598 = Or(x=w683, y=w682) -> (x .or. y?=w681:bool)
    n599 = global read "Robot Global Data.vi" "UDP Packet"() -> (w675:T12)
    n600 = Unbundle By Name(w675) -> ("Left Roller Pwr"=w674:dbl, "Right Roller Pwr"=w673:dbl)
    n601 = case shown="True" w717 {
      tunnel: [w1110 w1117] -> w801
      tunnel: [w1109 w1116] -> w711
      tunnel: w694 -> [w1108 w1115]
      tunnel: [w1105 w1114] -> w703
      tunnel: [w1107 w1113] -> w788
      tunnel: [w1106 w1112] -> w787
      tunnel: [w1104 w1111] -> w702
      frame False {
        # "Joystick"
        n602 = Unbundle By Name(w1108) -> ("Button 10"=w1107:bool, "Button 11"=w1106:bool, "Button 1"=w1110:bool, "Button 6"=w1109:bool, "Button 3"=w1105:bool, "Button 7"=w1104:bool)
      }
      frame True {
        # "Gamepad"
        n603 = Unbundle By Name(w1115) -> ("Button 10"=w1113:bool, "Button 9"=w1112:bool, "Button 5"=w1117:bool, "Button 8"=w1116:bool, "Button 2"=w1114:bool, "Button 7"=w1111:bool)
      }
    }
    n604 = And(x=w790, y=w761) -> (x .and. y?=w758:bool)
    n605 = And(x=w760, y=w761) -> (x .and. y?=w759:bool)
    n606 = Not(x=w651) -> (.not. x?=w647:bool)
    n607 = Or(x=w778, y=w758) -> (x .or. y?=w775:bool)
    n608 = Select(t=FALSE, s=w681, f=w792) -> (s? t:f=w650:bool)
    n609 = global read "Robot Global Data.vi" "UDP Packet"() -> (w657:T12)
    n610 = Unbundle By Name(w657) -> ("Shooting Delays"=w656:T45)
    n611 = case shown="False" w759 {
      tunnel: w758 -> [w889 _]
      tunnel: w757 -> [w888 _]
      tunnel: [w889 TRUE] -> w755
      tunnel: [w888 FALSE ("Elevator Active")] -> w756
      frame False {
      }
      frame True {
        # "2 Discs, reverse Right"
      }
    }
    n612 = Or(x=w777, y=w755) -> (x .or. y?=w776:bool)
    n613 = Or(x=w780, y=w756) -> (x .or. y?=w779:bool)
    n614 = Or(x=w782, y=w757) -> (x .or. y?=w781:bool)
    n615 = disable-structure shown="Disabled" {
      disable-tunnel: w788 -> [w840 _]
      disable-tunnel: w787 -> [w839 _]
      frame Disabled {
        # "Ratchet Locked state"
        # "Unlock Ratchet"
        # "Lock Ratchet"
        n616 = feedback #8(FALSE) -> (w833:bool)
        n617 = case shown="False" w840 {
          tunnel: w839 -> [w843 _]
          tunnel: [w842 TRUE] -> w831
          tunnel: w833 -> [w841 _]
          frame False {
            n618 = case shown="True" w843 {
              tunnel: [w844 FALSE] -> w842
              tunnel: w841 -> [w844 _]
              frame False {
              }
              frame True {
                # "Unlock"
              }
            }
          }
          frame True {
            # "Lock"
          }
        }
        n619 = feedback-in #8(w831) -> ()
        n620 = call <vilib>:"WPI_ServoRefNum Registry Get.vi"("refnum name"="Lock Servo") -> ("ServoDeviceRef"=w837:T46)  [unwired: 9 in, 1 out]
        n621 = Select(t=170.0, s=w831, f=0.0) -> (s? t:f=w836:dbl)
        n622 = call <vilib>:"SD Write Boolean.vi"("Boolean"=w831, "Name"="Lift/Ratchet Locked") -> ()  [unwired: 8 in, 2 out]
        n623 = call <vilib>:"WPI_ServoSetAngle.vi"("Angle"=w836, "ServoDeviceRef"=w837) -> ()  [unwired: 8 in, 2 out]
      }
      frame Enabled {
      }
    }
    n624 = And(x=w647, y=w650) -> (x .and. y?=w649:bool)
    n625 = global read "Robot Global Data.vi" "Azimuth Low Gear"() -> (w753:bool)
    n626 = global read "Robot Global Data.vi" "Encoder Values"() -> (w706:T41)
    n627 = Compound Arithmetic op=OR(w703, w702) -> (w704:bool)
    n628 = global read "Robot Global Data.vi" "Drive Controls"() -> (w705:T47)
    n629 = call <vilib>:"WPI_SolenoidRefNum Registry Get.vi"("refnum name"="Hopper Piston") -> ("SolenoidDevRef"=w785:T48)  [unwired: 9 in, 1 out]
    n630 = call "Motor Output.vi"("Max Power"=w674, "Backward"=w775, "Forward"=w781, "Motor refnum name"="Roller Front Left" ("refnum name")) -> ()  [unwired: 7 in, 1 out]
    n631 = call "Motor Output.vi"("Max Power"=w673, "Backward"=w776, "Forward"=w779, "Motor refnum name"="Roller Front Right" ("refnum name")) -> ()  [unwired: 7 in, 1 out]
    n632 = global read "Robot Global Data.vi" "UDP Packet"() -> (w708:T12)
    n633 = Unbundle By Name(w708) -> ("Auto Shift"=w707:T14)
    n634 = call "Flipper Delay.vi"("Shooting Delays"=w656, "RPM In Range"=w648, "Shoot Button"=w646, "Shoot Mode"=w649) -> ("Unjam Out"=w662:bool, "Flipper Out"=w729:bool)  [unwired: 6 in]
    n635 = call "Button Toggle.vi"("Button Input"=w801) -> ("Toggled Output"=w754:bool)  [unwired: 4 in]
    n636 = call-poly <vilib>:"WPI_SolenoidSet.vi"("Value"=w650, "SolenoidDevRef"=w785) -> ()  [unwired: 8 in, 2 out]
    n637 = call "Auto Shift.vi"("Auto Shift Settings"=w707, "Encoder Values"=w706, "Drive Controls"=w705) -> ("Low gear output"=w709:bool)  [unwired: 8 in]
    n638 = Unbundle By Name(w665) -> ("Manual Flipper"=w664:bool, "Manual Unjam"=w663:bool)
    n639 = Compound Arithmetic op=OR(w711, w681) -> (w680:bool)
    n640 = global read "Robot Global Data.vi" "Robot Mode"() -> (w748:T1)
    n641 = call <vilib>:"WPI_SolenoidRefNum Registry Get.vi"("refnum name"="Loader Ramp Piston") -> ("SolenoidDevRef"=w802:T48)  [unwired: 9 in, 1 out]
    n642 = call "Button Toggle.vi"("Button Input"=w704) -> ("Toggled Output"=w679:bool)  [unwired: 4 in]
    n643 = global read "Robot Global Data.vi" "Auton Commands"() -> (w639:T5)
    n644 = global read "Robot Global Data.vi" "Encoder Values"() -> (w672:T41)
    n645 = Unbundle By Name(w672) -> ("Avg Distance"=w670:dbl)
    n646 = call-poly <vilib>:"WPI_SolenoidSet.vi"("Value"=w680, "SolenoidDevRef"=w802) -> ()  [unwired: 8 in, 2 out]
    n647 = Equal?(x=WPI_DriverStationRobotMode2."Autonomous Enabled", y=w748) -> (x = y?=w745:bool)
    n648 = Or(x=w729, y=w664) -> (x .or. y?=w667:bool)
    n649 = call "Update Disc Count.vi"("Reset"=w768, "Manual Subtract"=w766, "Manual Add"=w767, "Disc IR Hopper"=w825, "Disc IR Shooter"=w824, "Flipper"=w667, "Disc Mode"=w692) -> ("Disc Count out"=w817:dbl)  [unwired: 4 in]
    n650 = call <vilib>:"SD Write Number.vi"("Numeric"=w817, "Name"="Sensor/Disc Count") -> ()  [unwired: 8 in, 2 out]
    n651 = global write "Robot Global Data.vi" "Disc Count"(w817) -> ()
    n652 = Or(x=w663, y=w662) -> (x .or. y?=w660:bool)
    n653 = Unbundle By Name(w639) -> ("Low Gear"=w744:bool)
    n654 = global read "Robot Global Data.vi" "UDP Packet"() -> (w671:T12)
    n655 = Unbundle By Name(w671) -> ("Toggle Ears Delay"=w668:dbl, "Toggle Ears Distance"=w669:dbl)
    n656 = And(x=w744, y=w745) -> (x .and. y?=w746:bool)
    n657 = global write "Robot Global Data.vi" "Drive Limit"(w680) -> ()
    n658 = call <vilib>:"SD Write Boolean.vi"("Boolean"=w680, "Name"="Auto/Load Ramp Down") -> ()  [unwired: 8 in, 2 out]
    n659 = global read "Robot Global Data.vi" "UDP Packet"() -> (w655:T12)
    n660 = Unbundle By Name(w655) -> ("Unjam Servo Angle"=w654:dbl)
    n661 = Compound Arithmetic op=OR(w746, w709, w754, w753) -> (w653:bool)
    n662 = call <vilib>:"WPI_SolenoidRefNum Registry Get.vi"("refnum name"="Flipper Piston") -> ("SolenoidDevRef"=w800:T48)  [unwired: 9 in, 1 out]
    n663 = global read "Robot Global Data.vi" "Robot Mode"() -> (w677:T1)
    n664 = call <vilib>:"WPI_SolenoidRefNum Registry Get.vi"("refnum name"="Gear Shifter") -> ("SolenoidDevRef"=w803:T48)  [unwired: 9 in, 1 out]
    n665 = call-poly <vilib>:"WPI_SolenoidSet.vi"("Value"=w667, "SolenoidDevRef"=w800) -> ()  [unwired: 8 in, 2 out]
    n666 = Not(x=w653) -> (.not. x?=w652:bool)
    n667 = call <vilib>:"WPI_ServoRefNum Registry Get.vi"("refnum name"="Unjam  Servo") -> ("ServoDeviceRef"=w661:T46)  [unwired: 9 in, 1 out]
    n668 = call "Toggle Lift Ears.vi"("Delay"=w668, "Distance Threshold"=w669, "Avg Distance"=w670, "Robot Mode"=w677) -> ("Lift Output"=w678:bool)  [unwired: 7 in]
    n669 = call-poly <vilib>:"WPI_SolenoidSet.vi"("Value"=w652, "SolenoidDevRef"=w803) -> ()  [unwired: 8 in, 2 out]
    n670 = call <vilib>:"WPI_SolenoidRefNum Registry Get.vi"("refnum name"="Lift Piston") -> ("SolenoidDevRef"=w799:T48)  [unwired: 9 in, 1 out]
    n671 = Select(t=w654, s=w660, f=0.0) -> (s? t:f=w659:dbl)
    n672 = call <vilib>:"WPI_SolenoidRefNum Registry Get.vi"("refnum name"="Low Gear Lights") -> ("SolenoidDevRef"=w716:T48)  [unwired: 9 in, 1 out]
    n673 = Or(x=w679, y=w678) -> (x .or. y?=w676:bool)
    n674 = call <vilib>:"WPI_ServoSetAngle.vi"("Angle"=w659, "ServoDeviceRef"=w661) -> ()  [unwired: 8 in, 2 out]
    n675 = call-poly <vilib>:"WPI_SolenoidSet.vi"("Value"=w653, "SolenoidDevRef"=w716) -> ()  [unwired: 8 in, 2 out]
    n676 = call-poly <vilib>:"WPI_SolenoidSet.vi"("Value"=w676, "SolenoidDevRef"=w799) -> ()  [unwired: 8 in, 2 out]
    n677 = Select(t=1.0, s=w653, f=2.0) -> (s? t:f=w771:dbl)
    n678 = call <vilib>:"SD Write Number.vi"("Numeric"=w771, "Name"="Drive/Gear") -> ()  [unwired: 8 in, 2 out]
  }
  "Feed Angle Ready" <- w1
  "Neutral Angle Ready" <- w1
